vi "AnalogDisc_Core.vi"(8 "error in":errorcluster, 9 "SignalBufferQueue in":refnum<queue>, 10 "DWFCtrlQueue in":refnum<queue>) -> (0 "error out":errorcluster)   [LabVIEW 2013, in "AnalogDiscSDKLv.lvlib"]
uses:
  <instrlib>/AnalogDiscSDKLv/AnalogDiscSDKLv.lvlib
  <instrlib>/AnalogDiscSDKLv/VIs/DWF_AnalogIn_Configurations.ctl
  <instrlib>/AnalogDiscSDKLv/VIs/DWF_AcqMode.ctl
  <instrlib>/AnalogDiscSDKLv/VIs/DWF_Filter.ctl
  <instrlib>/AnalogDiscSDKLv/VIs/DWF_TrigSrc.ctl
  <instrlib>/AnalogDiscSDKLv/VIs/DWF_TrigCond.ctl
  <instrlib>/AnalogDiscSDKLv/VIs/DWF_TrigType.ctl
  <instrlib>/AnalogDiscSDKLv/VIs/DWF_CtrlQueue.ctl
  <instrlib>/AnalogDiscSDKLv/VIs/DWF_State.ctl
  <instrlib>/AnalogDiscSDKLv/VIs/DWF_PrivateStats.ctl
  <instrlib>/AnalogDiscSDKLv/VIs/DWF_InstrumentStatus.ctl
  <instrlib>/AnalogDiscSDKLv/VIs/DWF_DwfState.ctl
  <instrlib>/AnalogDiscSDKLv/VIs/DWF_Signal.ctl
  <instrlib>/AnalogDiscSDKLv/VIs/DWF_TrigLen.ctl
  <instrlib>/AnalogDiscSDKLv/VIs/DWF_DWFERC.ctl
  <vilib>/Utility/error.llb/DialogType.ctl
  <instrlib>/AnalogDiscSDKLv/VIs/DWF_AnalogOut_ChannelConfigurations.ctl
  <instrlib>/AnalogDiscSDKLv/VIs/DWF_Function.ctl
  <instrlib>/AnalogDiscSDKLv/VIs/DWF_Node.ctl
  <vilib>/Utility/miscctls.llb/LVPositionTypeDef.ctl
  <vilib>/Analysis/1siggen.llb/Ramp Pattern by Samples.vi
  <vilib>/Utility/error.llb/Error Cluster From Error Code.vi
  <vilib>/ErrorRing/Error Ring.xnode
  <vilib>/ptbypt/NI_PtbyPt.lvlib
  <userlib>/Utility/ErrorLog_lib.lvlib
  Windows/System32/dwf.dll
  <vilib>/Analysis/NI_AALBase.lvlib
panel:
  out "WaitForVoltageStablize":bool
  in  "GetInfo":bool
  out "psecPosition":dbl
  out "elements":T1[](array[typedef])
  out "sysCount_inPCTrig":i32
  out "PCTrig_counter":i32
  out "AO2_sts":T3=enum."Armed"
  out "AO1_sts":T3=enum."Armed"
  in  "fStart_AO":bool
  in  "SetFuncData_AO":bool
  in  "SetTrigSrc_AO":bool
  in  "SetEnable_AO":bool
  in  "SetConfig_AO":bool
  in  "SetStates_AO":bool
  out "waited t PCTrig":u32
  out "AI_sts":T4
  in  "TriggerPC":bool
  out "Live Stats":T5
  in  "Mode(N/T)":bool caption="Mode"
  out "Graph":sgl[][](graph)
  in  "fConfig":bool
  in  "Reset":bool
  in  "CloseAll":bool
  in  "Close":bool
  in  "Enumerate":bool
  in  "Open":bool
  in  "Quit":bool
  in  "Start":bool
  in  "ConfigAll":bool
  out "UserName":string[](array[string])
  out "SN":string[](array[string])
  out "DevName":string[](array[string])
  out "DeviceID":i32[](array[numeric])
  out "pnDevice":i32
  out "isBusy":i32[](array[numeric])
  out "DeviceVersion":i32[](array[numeric])
  in  "Configurations":T6={"Acqusition"={"Freq(Hz,SampleRate)"=10000000.0, "BufferSize"=8192, "Mode"=enum."Single", "RecordLength(s)"=0.0008192}, "Channels"=[{"Range(V)"=5.0, "Offset(V)"=0.0, "Filter"=enum."Decimate", "Enable"=TRUE}], "Trigger"={"TriggerSource"=enum."None", "Timeout(s)"=0.0, "Holdoff(s)"=1e-06, "Position/Delay(s)"=0.0}, "AnalogTrigger"={"Channel"=0, "Polarity"=enum."Rising", "Type"=enum."Pulse", "Level(V)"=0.0, "Filter"=enum."MinMax", "Hysterisis(V)"=0.0}, "DevSN"="-1"} {"AnalogTrigger"."Channel" format="%#_6p"; "AnalogTrigger"."Hysterisis(V)" format="%#_6p"; "Acqusition"."RecordLength(s)" format="%#_6p"; "Acqusition"."Freq(Hz,SampleRate)" format="%#_6p"; "Acqusition"."BufferSize" min=1 max=16384 step=1; "Trigger"."Position/Delay(s)" format="%#_6p"; "Trigger"."Holdoff(s)" format="%#_6p"}
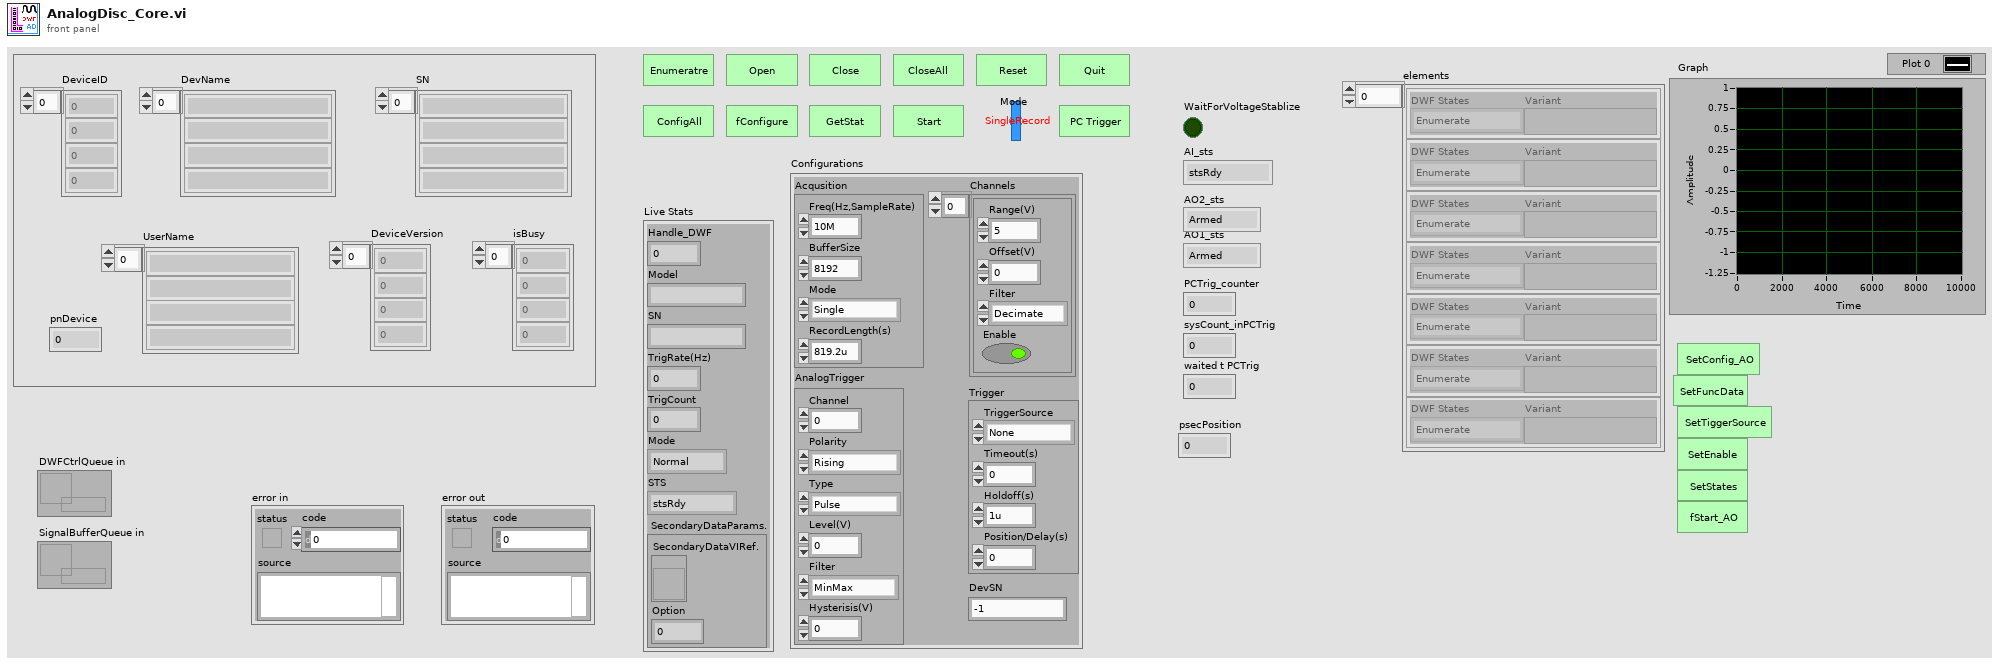
[diagram p1: front panel]
types:
  T1 = typedef "AnalogDiscSDKLv.lvlib/DWF_CtrlQueue.ctl" = cluster{"DWF States":T2, "Variant":variant}
  T2 = typedef "AnalogDiscSDKLv.lvlib/DWF_State.ctl" = enum16{"Enumerate", "Open", "Close", "CloseAll", "Reset", "Quit", "==Settings==", "SetAcquisition_", "SetChannels_", "SetTrigger_", "SetAnalogTrigDetector_", "SetAll_AcquChTrig_", "fConfigurate", "fStart", "GetStatus", "_WaitForDone/Idle", "_GetData", "GetAcquisition", "GetChannels", "GetTrigger", "GetAll_AcquChTrig", "==Messaging==", "_PushDataOut", "GetStat_", "GetConfig_", "==ModeSetup==", "SetSignalBuffer_", "SetMode_", "SetSecondaryDataRef._", "==AnalogOut==", "GetChannelCount_AO", "fStart_AO", "SetChEnable_AO", "SetConfig_AO", "SetFuncData_AO", "SetOffset_AO_", "SetMasterNode_AO", "SetStates_AO", "SetSymetry_AO", "SetTriggerSource_AO", "==Trigger==", "ManualTrigger"}
  T3 = typedef "AnalogDiscSDKLv.lvlib/DWF_DwfState.ctl" = enum16{"Ready", "Armed", "Done", "Running", "Config", "Prefill", "---", "Wait"}
  T4 = typedef "AnalogDiscSDKLv.lvlib/DWF_InstrumentStatus.ctl" = enum16{"stsRdy", "stsARM", "stsDone", "stsTrig", "stsCfg", "stsPrefill", "stsNotDone", "stsTrigDly", "stsError", "stsBusy", "stsStop"}
  T5 = typedef "AnalogDiscSDKLv.lvlib/DWF_PrivateStats.ctl" = cluster{"Handle_DWF":i32, "Model":string, "SN":string, "TrigRate(Hz)":dbl, "TrigCount":i32, "Mode":enum16{"Normal", "Turbo"}, "STS":T4, "SecondaryDataParams.":cluster{"SecondaryDataVIRef.":refnum<vi>, "Option":i32}}
  T6 = typedef "AnalogDiscSDKLv.lvlib/DWF_AnalogIn_Configurations.ctl" = cluster{"Acqusition":cluster{"Freq(Hz,SampleRate)":dbl, "BufferSize":i32, "Mode":T7, "RecordLength(s)":dbl}, "Channels":cluster{"Range(V)":dbl, "Offset(V)":dbl, "Filter":T8, "Enable":bool}[], "Trigger":cluster{"TriggerSource":T9, "Timeout(s)":dbl, "Holdoff(s)":dbl, "Position/Delay(s)":dbl}, "AnalogTrigger":cluster{"Channel":i32, "Polarity":T10, "Type":T11, "Level(V)":dbl, "Filter":T8, "Hysterisis(V)":dbl}, "DevSN":string}
  T7 = typedef "AnalogDiscSDKLv.lvlib/DWF_AcqMode.ctl" = enum16{"Single", "ScanShift", "ScanScreen", "Record"}
  T8 = typedef "AnalogDiscSDKLv.lvlib/DWF_Filter.ctl" = enum16{"Decimate", "Average", "MinMax"}
  T9 = typedef "AnalogDiscSDKLv.lvlib/DWF_TrigSrc.ctl" = enum16{"None", "PC", "DetectorAnalogIn", "DetectorDigitalIn", "AnalogIn", "DigitalIn", "DigitalOut", "AnalogOut1", "AnalogOut2", "AnalogOut3", "AnalogOut4", "External1", "External2", "External3", "External4"}
  T10 = typedef "AnalogDiscSDKLv.lvlib/DWF_TrigCond.ctl" = enum16{"Rising", "Falling"}
  T11 = typedef "AnalogDiscSDKLv.lvlib/DWF_TrigType.ctl" = enum16{"Edge", "Pulse", "Transition"}
  T12 = typedef "LVPositionTypeDef.ctl" = cluster{"Left":i32, "Top":i32}
  T13 = typedef "AnalogDiscSDKLv.lvlib/DWF_AnalogOut_ChannelConfigurations.ctl" = cluster{"FUNC":T14, "Frequency(Hz)_AO":dbl, "Amplitude(V)_AO":dbl, "Phase(deg)_AO":dbl, "Offset(V)_AO":dbl, "rgdData":dbl[], "cData":i32, "Symmetry":dbl, "Enable":bool, "Node":T15}
  T14 = typedef "AnalogDiscSDKLv.lvlib/DWF_Function.ctl" = u8
  T15 = typedef "AnalogDiscSDKLv.lvlib/DWF_Node.ctl" = enum16{"Carrier", "FM", "AM"}
  T16 = cluster{"Configs":T13[], "ChannelCount":i32, "States":cluster{"Wait(s)":dbl, "Run(s)":dbl, "cRepeat":i32, "TriggerSource":T9}[]}
  T17 = typedef "DialogType.ctl" = u16
  T18 = typedef "AnalogDiscSDKLv.lvlib/DWF_DWFERC.ctl" = enum16{"dwfercNoErc", "dwfercUnknownError", "dwfercApiLockTimeout", "dwfercAlreadyOpened", "dwfercNotSupported", "dwfercInvalidParameter0", "dwfercInvalidParameter1", "dwfercInvalidParameter2", "dwfercInvalidParameter3"}
  T19 = typedef "AnalogDiscSDKLv.lvlib/DWF_TrigLen.ctl" = enum16{"triglenLess", "triglenTimeout", "triglenMore"}
  T20 = typedef "AnalogDiscSDKLv.lvlib/DWF_Signal.ctl" = cluster{"tickcount":u32, "Signal":sgl[][], "SecondaryData":dbl[]}
  T21 = cluster{"Freq(Hz,SampleRate)":dbl, "BufferSize":i32, "Mode":T7, "RecordLength(s)":dbl}
  T22 = cluster{"Range(V)":dbl, "Offset(V)":dbl, "Filter":T8, "Enable":bool}[]
  T23 = cluster{"TriggerSource":T9, "Timeout(s)":dbl, "Holdoff(s)":dbl, "Position/Delay(s)":dbl}
  T24 = cluster{"Channel":i32, "Polarity":T10, "Type":T11, "Level(V)":dbl, "Filter":T8, "Hysterisis(V)":dbl}
  T25 = cluster{"SecondaryDataVIRef.":refnum<vi>, "Option":i32}
  T26 = cluster{"Wait(s)":dbl, "Run(s)":dbl, "cRepeat":i32, "TriggerSource":T9}[]
  T27 = cluster{"Wait(s)":dbl, "Run(s)":dbl, "cRepeat":i32, "TriggerSource":T9}
  T28 = cluster{i32, "States":cluster{"Wait(s)":dbl, "Run(s)":dbl, "cRepeat":i32, "TriggerSource":T9}}
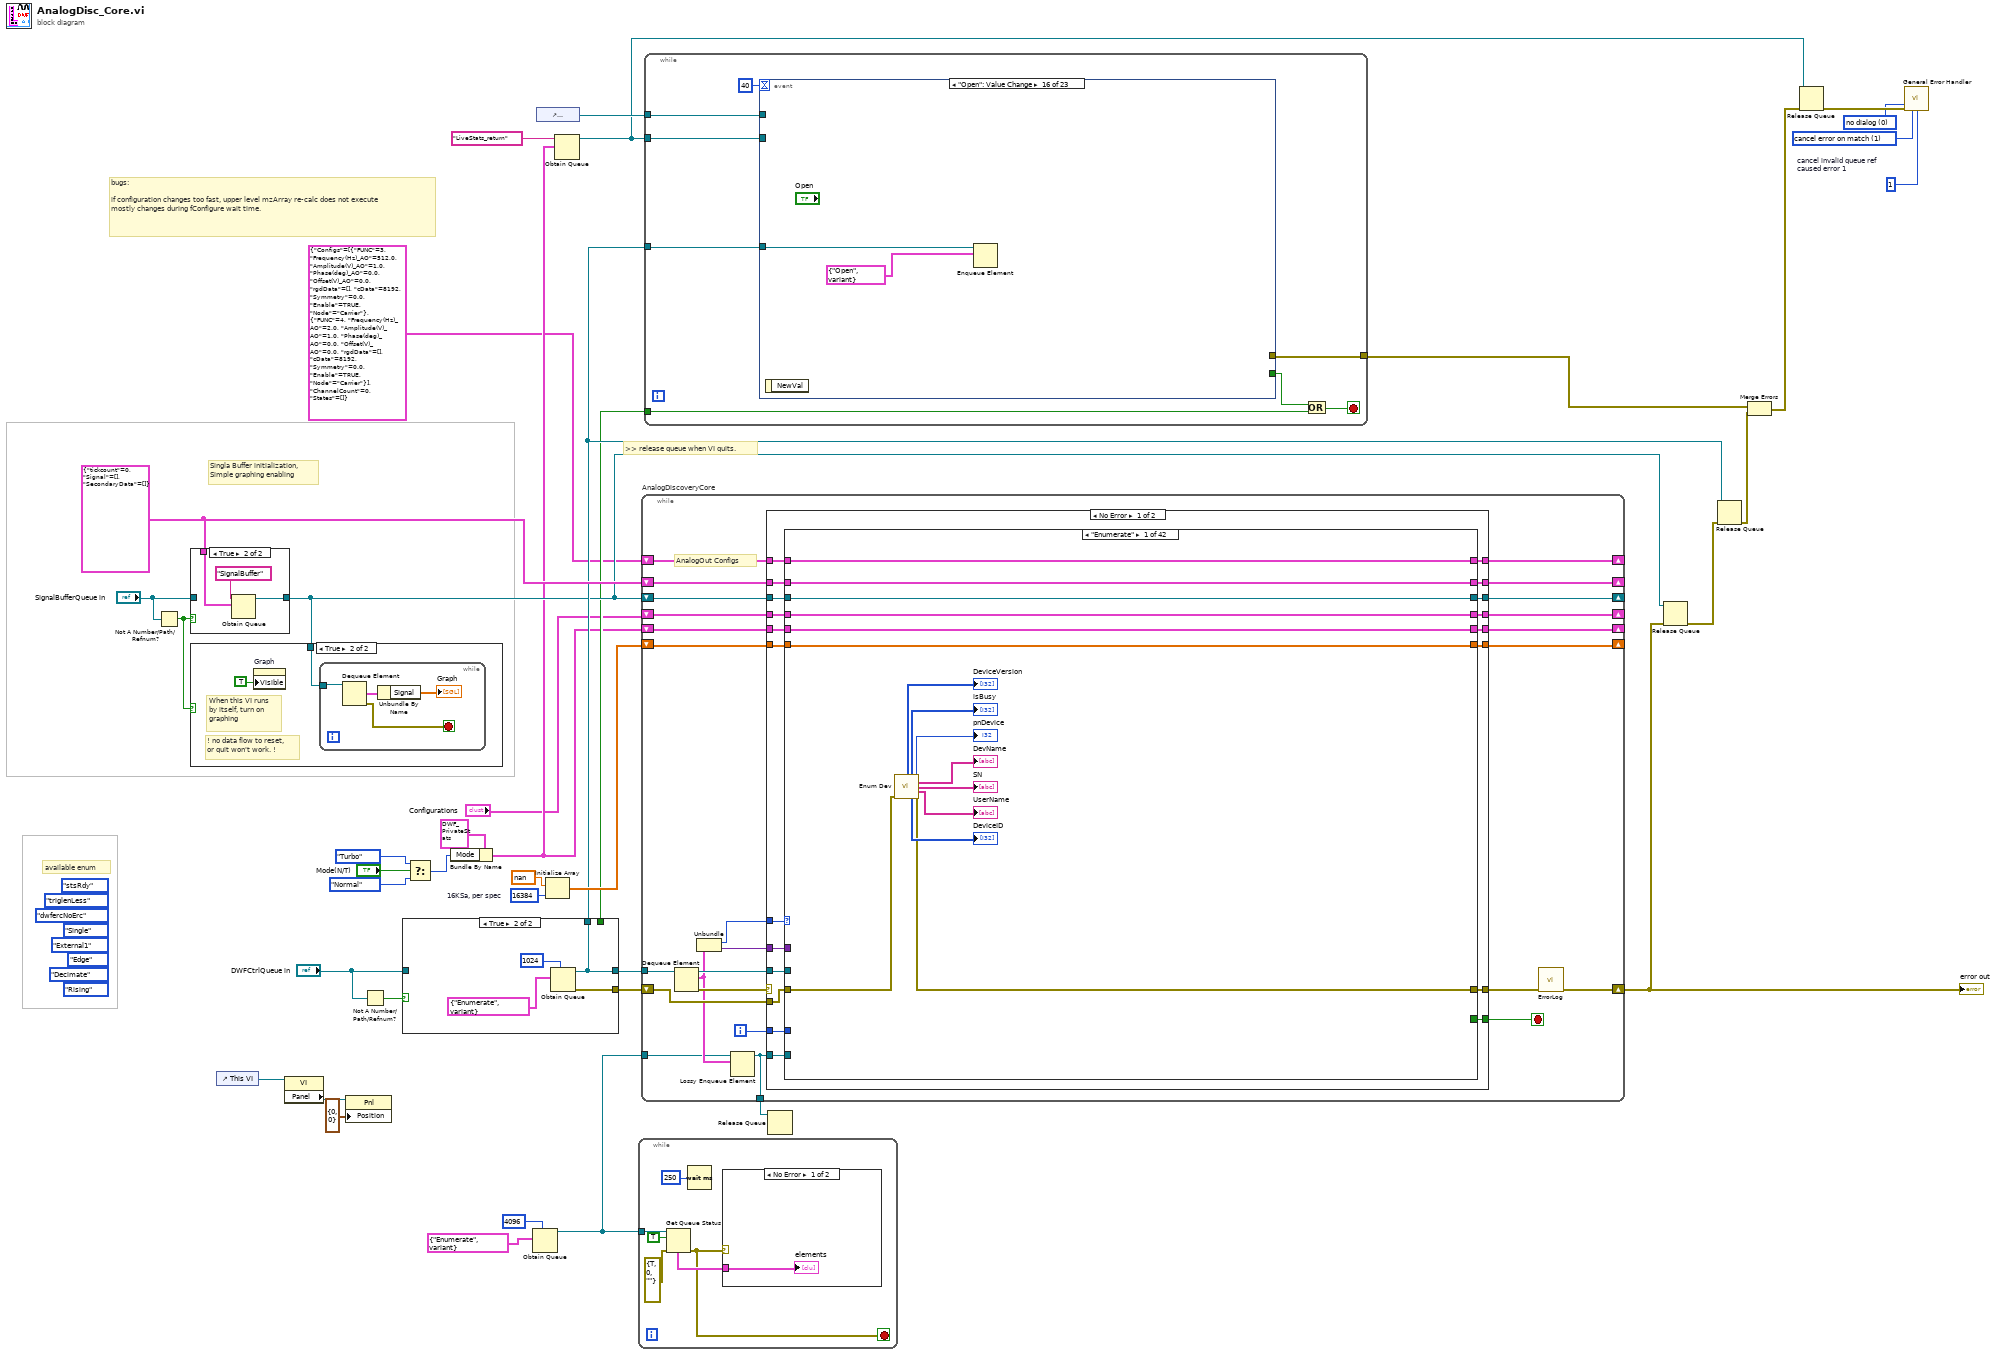
[diagram p0: block diagram]
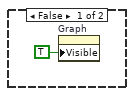
[diagram p3: hidden frame]
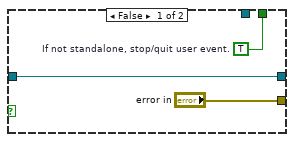
[diagram p5: hidden frame]
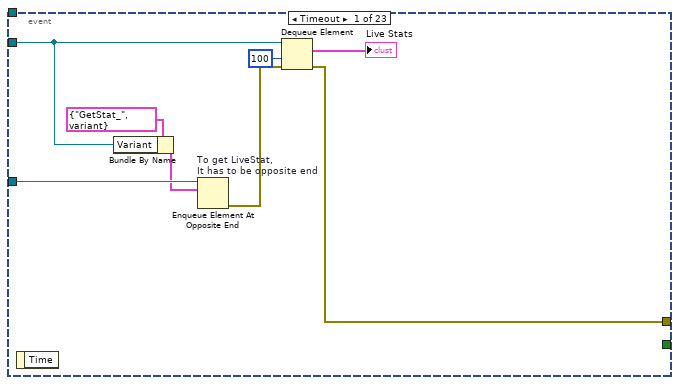
[diagram p6: hidden frame]
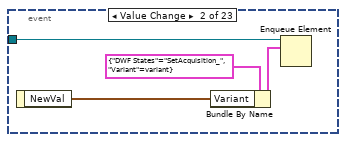
[diagram p7: hidden frame]
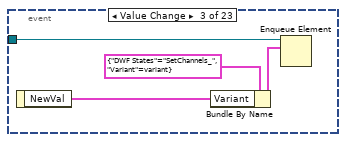
[diagram p8: hidden frame]
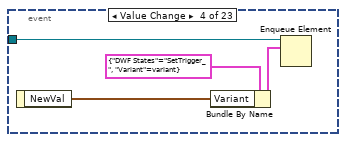
[diagram p9: hidden frame]
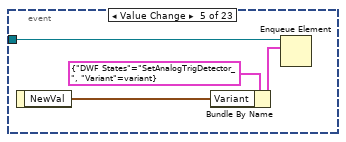
[diagram p10: hidden frame]
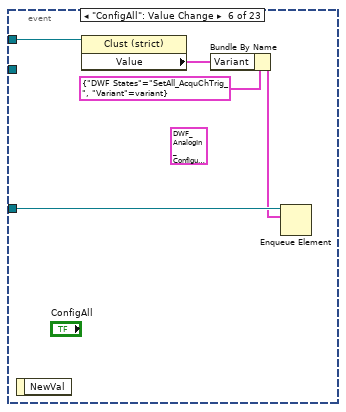
[diagram p11: hidden frame]
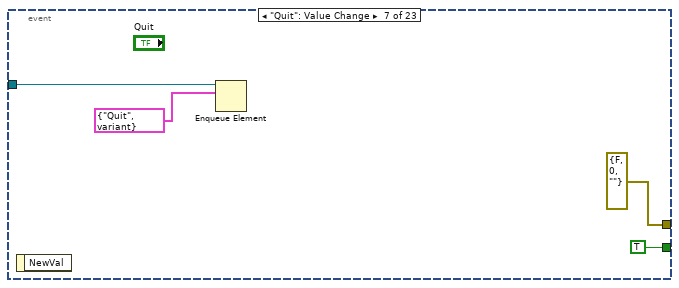
[diagram p12: hidden frame]
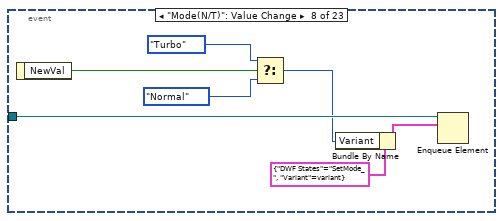
[diagram p13: hidden frame]
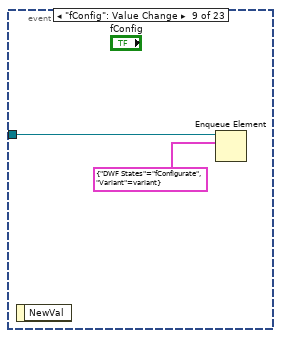
[diagram p14: hidden frame]
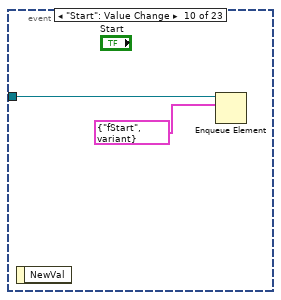
[diagram p15: hidden frame]
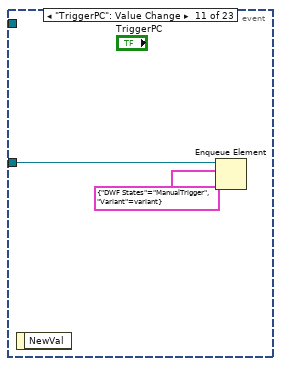
[diagram p16: hidden frame]
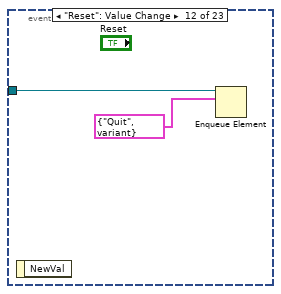
[diagram p17: hidden frame]
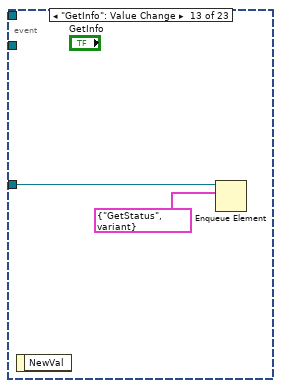
[diagram p18: hidden frame]
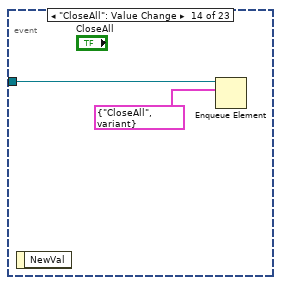
[diagram p19: hidden frame]
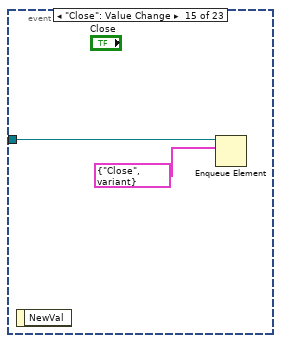
[diagram p20: hidden frame]
diagram:
  w19 = 1  # cancel invalid queue ref caused error 1
  w20 = 1 items=["no exception", "cancel error on match", "set error on match"] ("[exception action] (none:0)")
  w21 = T17 0 items=["no dialog", "OK message", "continue or stop message", "OK message + warnings", "continue/stop + warnings"] ("type of dialog (OK msg:1)")
  (unwired) DWF_TrigSrc."External1" ("TriggerSource")
  (unwired) DWF_DWFERC."dwfercNoErc" ("DWFErC")
  (unwired) DWF_TrigLen."triglenLess" ("TrigLen")
  (unwired) DWF_TrigCond."Rising" ("TrigCond")
  (unwired) DWF_TrigType."Edge" ("TrigType")
  (unwired) DWF_Filter."Decimate" ("Filter")
  (unwired) DWF_AcqMode."Single" ("ACQMODE")
  (unwired) DWF_InstrumentStatus."stsRdy" ("STS")
  w38 = 16384  # 16KSa, per spec
  w40 = T20 {"tickcount"=0, "Signal"=[], "SecondaryData"=[]} ("Signal_Typedef")
  # "bugs:\n\nif configuration changes too fast, upper level mzArray re-calc does not execute\nmostly changes during fConfigure wait time."
  # "Singla Buffer initialization,\nSimple graphing enabling"
  # "available enum"
  # ">> release queue when VI quits."
  n1 = Not A Number/Path/Refnum?(number/path/refnum="SignalBufferQueue in") -> (NaN/Path/Refnum?=w24:bool)
  n2 = case shown="True" w24 {
    tunnel: w40 -> [_ w44]
    tunnel: [w41 w43] -> w25
    tunnel: "SignalBufferQueue in" -> [w41 _]
    frame False {
    }
    frame True {
      n3 = Obtain Queue(name (unnamed)="SignalBuffer", element data type=w44) -> (queue out=w43:refnum<queue>)  [unwired: 3 in, 2 out]
    }
  }
  n4 = case shown="True" w24 {
    tunnel: w25 -> [_ w47]
    frame False {
      n5 = property on="Graph" class="WFGraph (strict)"("Visible"=TRUE) -> ()  [unwired: 2 in, 2 out]
    }
    frame True {
      # "! no data flow to reset,\nor quit won't work. !"
      # "When this VI runs\nby itself, turn on \ngraphing"
      n6 = property on="Graph" class="WFGraph (strict)"("Visible"=TRUE) -> ()  [unwired: 2 in, 2 out]
      n7 = while {
        tunnel: w47 -> [w51]
        stop <- w48 stop-if-true
        n8 = Dequeue Element(queue=w51) -> (element=w50:T20, error out=w48:errorcluster)  [unwired: 2 in, 2 out]
        n9 = Unbundle By Name(w50) -> ("Signal"=→"Graph":sgl[][])
      }
    }
  }
  n10 = control-ref of="This VI"() -> (w3:refnum<vi>)
  n11 = property class="VI"(reference=w3) -> ("Panel"=w2:refnum<vi>)  [unwired: 1 in, 2 out]
  n12 = property class="Pnl"(reference=w2, "Position"=T12 {"Left"=0, "Top"=0}) -> ()  [unwired: 1 in, 2 out]
  n13 = Not A Number/Path/Refnum?(number/path/refnum="DWFCtrlQueue in") -> (NaN/Path/Refnum?=w34:bool)
  n14 = case shown="True" w34 {
    tunnel: [w54 w55] -> w36
    tunnel: ["error in" w58] -> w35
    tunnel: "DWFCtrlQueue in" -> [w54 _]
    tunnel: [_ w55] -> w30
    tunnel: [w52 _] -> w18
    frame False {
      w52 = TRUE  # If not standalone, stop/quit user event.
    }
    frame True {
      n15 = Obtain Queue(max queue size (-1, unlimited)=1024, element data type=T1 {"DWF States"=enum."Enumerate", "Variant"=variant}) -> (queue out=w55:refnum<queue>, error out=w58:errorcluster)  [unwired: 3 in, 1 out]
    }
  }
  n16 = Select(t=enum16{"Normal", "Turbo"}."Turbo" ("Mode"), s="Mode(N/T)", f=enum16{"Normal", "Turbo"}."Normal" ("Mode")) -> (s? t:f=w11:enum16{"Normal", "Turbo"})
  n17 = Bundle By Name(cluster=T5 {"Handle_DWF"=0, "Model"="", "SN"="", "TrigRate(Hz)"=0.0, "TrigCount"=0, "Mode"=enum."Normal", "STS"=enum."stsRdy", "SecondaryDataParams."={"SecondaryDataVIRef."=refnum, "Option"=0}} ("PrivateStats(Live)"), "Mode"=w11) -> (w15:T5)
  n18 = Obtain Queue(max queue size (-1, unlimited)=4096, element data type=T1 {"DWF States"=enum."Enumerate", "Variant"=variant}) -> (queue out=w5:refnum<queue>)  [unwired: 3 in, 2 out]
  n19 = control-ref of="Configurations"() -> (w32:refnum<vi>)
  n20 = Initialize Array(nan ("Numeric"), w38) -> (w37:dbl[])
  n21 = Obtain Queue(name (unnamed)="LiveStats_return", element data type=w15) -> (queue out=w28:refnum<queue>)  [unwired: 3 in, 2 out]
  n22 = while {
    tunnel: w5 -> [w64]
    stop <- w61 stop-if-true
    n23 = Get Queue Status(queue=w64, return elements? (F)=TRUE, error in (no error)=errorcluster {"status"=TRUE, "code"=0, "source"=""}) -> (error out=w61:errorcluster, elements=w62:T1[])  [unwired: 6 out]
    n24 = Wait (ms)(milliseconds to wait=u32 250) -> ()  [unwired: 1 out]
    n25 = case shown="No Error" w61 {
      tunnel: w62 -> [w65 _]
      frame No Error {
        "elements" <- w65
      }
      frame Error {
      }
    }
  }
  n26 = while "AnalogDiscoveryCore" {
    shift-right: [w89] -> _
    shift-left: w25 -> [w90]
    tunnel: w36 -> [w71]
    shift-right: [w70] -> w23
    shift-left: w35 -> [w77]
    shift-right: [w86] -> _
    shift-left: "Configurations" -> [w85]
    shift-right: [w78] -> _
    shift-left: w15 -> [w84]
    shift-right: [w79] -> _
    shift-left: w37 -> [w82]
    shift-right: [w80] -> _
    shift-left: w40 -> [w83]
    shift-right: [w73] -> _
    shift-left: T16 {"Configs"=[{"FUNC"=3, "Frequency(Hz)_AO"=512.0, "Amplitude(V)_AO"=1.0, "Phase(deg)_AO"=0.0, "Offset(V)_AO"=0.0, "rgdData"=[], "cData"=8192, "Symmetry"=0.0, "Enable"=TRUE, "Node"=enum."Carrier"}, {"FUNC"=4, "Frequency(Hz)_AO"=2.0, "Amplitude(V)_AO"=1.0, "Phase(deg)_AO"=0.0, "Offset(V)_AO"=0.0, "rgdData"=[], "cData"=8192, "Symmetry"=0.0, "Enable"=TRUE, "Node"=enum."Carrier"}], "ChannelCount"=0, "States"=[]} -> [w74]
    tunnel: w5 -> [w68]
    tunnel: [w66] -> w4
    i -> [w72]
    stop <- w88 stop-if-true
    # "AnalogOut Configs"
    n27 = Dequeue Element(queue=w71) -> (queue out=w75:refnum<queue>, element=w69:T1, error out=w76:errorcluster)  [unwired: 2 in, 1 out]
    n28 = Unbundle(w69) -> ("DWF States"=w67:T2, "Variant"=w81:variant)
    n29 = Lossy Enqueue Element(queue=w68, element=w69) -> (queue out=w66:refnum<queue>)  [unwired: 1 in, 3 out]
    n30 = case shown="No Error" w76 {
      tunnel: w90 -> [w110 w1205]
      tunnel: [w109 w1205] -> w89
      tunnel: [w108 TRUE] -> w88
      tunnel: [w107 w1203] -> w87
      tunnel: [w106 w1206] -> w86
      tunnel: w85 -> [w105 w1206]
      tunnel: w84 -> [w104 w1207]
      tunnel: w83 -> [w103 w1204]
      tunnel: w82 -> [w102 w1208]
      tunnel: w75 -> [w101 _]
      tunnel: w67 -> [w100 _]
      tunnel: w81 -> [w99 _]
      tunnel: [w98 w1204] -> w80
      tunnel: [w97 w1208] -> w79
      tunnel: [w96 w1207] -> w78
      tunnel: w77 -> [w95 _]
      tunnel: w74 -> [w94 w1202]
      tunnel: [w93 w1202] -> w73
      tunnel: w72 -> [w92 _]
      tunnel: w66 -> [w91 _]
      frame No Error {
        n31 = case shown="\"Enumerate\"" w100 {
          tunnel: w110 -> [w125 w139 w184 w192 w208 w224 w248 w267 w301 w337 w367 w396 w440 w456 w469 w493 w559 w586 w593 w600 w612 w624 w631 w675 w687 w699 w708 w743 w767 w774 w785 w800 w828 w872 w933 w978 w1020 w1069 w1117 w1153 w1160 w1181]
          tunnel: [w125 w139 w184 w192 w208 w224 w248 w267 w301 w337 w367 w396 w440 w456 w469 w493 w559 w586 w593 w600 w612 w624 w631 w675 w687 w699 w708 w744 w767 w774 w785 w800 w828 w872 w933 w978 w1020 w1069 w1117 w1153 w1160 w1181] -> w109
          tunnel: [_ _ _ _ _ w218 _ _ _ _ _ _ _ _ _ _ _ _ _ _ _ _ _ _ _ _ _ _ _ _ _ _ _ _ _ _ _ _ _ _ _ _] -> w108
          tunnel: w101 -> [_ _ _ _ w204 w215 _ _ _ _ _ w392 _ w443 _ w495 w547 _ _ _ _ _ w647 _ _ _ _ _ _ _ _ _ _ _ _ _ _ _ _ _ _ _]
          tunnel: w95 -> [w116 _ w176 w191 w203 w216 _ w258 w292 w329 w360 w386 w433 w447 w463 w494 w545 w585 w592 w599 w602 _ w649 w669 w677 _ w713 w740 w756 w773 w775 w787 w818 w863 w924 w969 w1011 w1060 w1102 w1147 _ w1174]
          tunnel: [w117 w134 w175 w191 w202 w217 w243 w259 w293 w326 w357 w391 w427 w449 w462 w487 w549 w585 w592 w599 w603 w619 w648 w668 w678 w694 w709 w741 w757 w773 w776 w788 w819 w864 w925 w970 w1012 w1061 w1109 w1142 w1154 w1175] -> w107
          tunnel: [w124 w132 w183 w190 w207 w223 w247 w264 w298 w334 w364 w389 w439 w455 w468 w492 w564 w584 w591 w598 w604 w623 w651 w667 w679 w698 w717 w749 w766 w772 w784 w799 w827 w871 w932 w977 w1019 w1068 w1116 w1152 w1159 w1180] -> w106
          tunnel: w105 -> [w124 w132 w183 w190 w207 w223 w247 w262 w296 w332 w362 w389 w439 w455 w468 w492 w564 w584 w591 w598 w604 w623 w651 w667 w679 w698 w717 w749 w766 w772 w784 w799 w827 w871 w932 w977 w1019 w1068 w1116 w1152 w1159 w1180]
          tunnel: [w123 w137 w179 w189 w201 w220 w246 w265 w299 w335 w365 w395 w435 w451 w461 w484 w542 w583 w590 w597 w611 w622 w645 w666 w686 w697 w710 w748 w763 w771 w780 w796 w824 w868 w929 w974 w1016 w1065 w1113 w1149 w1158 w1176] -> w96
          tunnel: w104 -> [w123 w136 w180 w189 w201 w220 w246 w265 w299 w335 w365 w395 w435 w451 w465 w485 w552 w583 w590 w597 w611 w622 w635 w666 w686 w697 w707 w748 w762 w771 w780 w796 w824 w868 w929 w974 w1016 w1065 w1113 w1149 w1158 w1176]
          tunnel: w103 -> [w122 w138 w182 w188 w206 w222 w245 w266 w300 w336 w366 w394 w438 w454 w467 w490 w558 w582 w589 w596 w610 w621 w644 w674 w685 w696 w716 w747 w765 w770 w783 w798 w826 w870 w931 w976 w1018 w1067 w1115 w1151 w1157 w1179]
          tunnel: w102 -> [w115 w135 w177 w187 w205 w221 w244 w255 w290 w327 w358 w393 w432 w445 w466 w486 w563 w581 w588 w595 w609 w620 w646 w673 w684 w695 w715 w746 w764 w769 w782 w797 w825 w869 w930 w975 w1017 w1066 w1114 w1150 w1156 w1178]
          tunnel: w99 -> [_ _ _ _ _ _ _ w263 w297 w333 w363 w390 _ _ _ _ _ _ _ _ w608 _ _ w670 w683 _ w714 w745 w761 _ _ w794 w822 w866 w927 w972 w1014 w1063 w1111 w1148 _ _]
          tunnel: [w122 w138 w182 w188 w206 w222 w245 w266 w300 w336 w366 w394 w438 w454 w467 w490 w557 w582 w589 w596 w610 w621 w644 w674 w685 w696 w716 w747 w765 w770 w783 w798 w826 w870 w931 w976 w1018 w1067 w1115 w1151 w1157 w1179] -> w98
          tunnel: [w115 w135 w177 w187 w205 w221 w244 w256 w290 w327 w358 w393 w432 w445 w466 w486 w543 w581 w588 w595 w609 w620 w646 w673 w684 w695 w715 w746 w764 w769 w782 w797 w825 w869 w930 w975 w1017 w1066 w1114 w1150 w1156 w1178] -> w97
          tunnel: w94 -> [w111 w133 w174 w185 w195 w213 w242 w254 w289 w325 w356 w385 w431 w444 w459 w471 w539 w580 w587 w594 w601 w618 w634 w664 w676 w693 w705 w737 w755 w768 w781 w793 w816 w857 w918 w963 w1005 w1056 w1105 w1141 w1155 w1177]
          tunnel: [w111 w133 w174 w185 w195 w213 w242 w254 w289 w325 w356 w385 w431 w444 w459 w471 w539 w580 w587 w594 w601 w618 w634 w664 w676 w693 w705 w737 w755 w768 w778 w793 w815 w856 w917 w962 w1004 w1055 w1104 w1141 w1155 w1177] -> w93
          tunnel: w92 -> [_ _ _ _ _ _ _ _ _ _ _ _ _ _ _ _ _ _ _ _ _ _ _ _ _ _ _ _ _ _ _ _ _ _ _ _ _ _ _ _ _ w1166]
          tunnel: w91 -> [_ _ _ _ _ _ _ _ _ _ _ _ _ _ _ _ _ _ _ _ _ _ _ _ _ _ _ _ _ _ _ _ _ _ _ _ _ _ _ _ _ _]
          frame "Enumerate" {
            n32 = call <instrlib>:"Enum Dev.vi"("error in (no error)"=w116) -> ("DeviceVersion"=→"DeviceVersion":i32[], "isBusy"=→"isBusy":i32[], "pnDevice"=→"pnDevice":i32, "DevName"=→"DevName":string[], "SN"=→"SN":string[], "UserName"=→"UserName":string[], "DeviceID"=→"DeviceID":i32[], "error out"=w117:errorcluster)  [unwired: 7 in]
          }
          frame "Open" {
            # "if did not fine => -1,\nwhich mean the first\navailable device."
            n33 = Unbundle By Name(w132) -> ("DevSN"=w126:string)
            n34 = call <instrlib>:"Enum Dev.vi"() -> ("DevName"=w129:string[], "SN"=w131:string[], "error out"=w130:errorcluster)  [unwired: 8 in, 5 out]
            n35 = Search 1D Array "find index of the dev by SN"(1D array=w131, element=w126) -> (index of element=w127:i32)  [unwired: 1 in]
            n36 = Less Than 0?(x=w127) -> (x < 0?=w128:bool)
            n37 = case shown="False" w128 {
              tunnel: [w149 w167] -> w137
              tunnel: w136 -> [w148 w167]
              tunnel: [w145 w168] -> w134
              tunnel: w130 -> [w143 _]
              tunnel: w126 -> [w142 _]
              tunnel: w129 -> [w141 _]
              tunnel: w127 -> [w140 _]
              frame False {
                n38 = call <vilib>:"Clear Errors.vi"("error in (no error)"=w143) -> ("error out"=w146:errorcluster)  [unwired: 6 in]
                n39 = call <instrlib>:"Open Dev.vi"("error in (no error)"=w146, "idxDev"=w140) -> ("error out"=w147:errorcluster, "hdwf"=w144:i32)  [unwired: 7 in, 1 out]
                n40 = case shown="No Error" w147 {
                  selector: w147 -> [w153 _]
                  tunnel: [w159 w161] -> w149
                  tunnel: w144 -> [w156 _]
                  tunnel: w148 -> [w155 w161]
                  tunnel: w142 -> [w154 _]
                  tunnel: [w153 w160] -> w145
                  tunnel: w141 -> [w152 _]
                  tunnel: w140 -> [w150 _]
                  frame No Error {
                    n41 = Index Array(array=w152, index=w150) -> (element=w151:string)
                    n42 = Bundle By Name(cluster=w155, "Handle_DWF"=w156, "SN"=w154, "TrigRate(Hz)"=0.0, "TrigCount"=0, "Model"=w151) -> (w159:T5)
                  }
                  frame Error {
                    n43 = xnode "Error Ring"() -> ("error out"=w160:errorcluster)
                  }
                }
              }
              frame True {
                n44 = xnode "Error Ring"() -> ("error out"=w168:errorcluster)
              }
            }
          }
          frame "Close" {
            n45 = Unbundle By Name(w180) -> ("Handle_DWF"=w181:i32)
            n46 = call <instrlib>:"Close Dev.vi"("error in (no error)"=w176, "hdwf"=w181) -> ("error out"=w175:errorcluster)  [unwired: 8 in, 1 out]
            n47 = Bundle By Name(cluster=w180, "Handle_DWF"=-1) -> (w179:T5)
          }
          frame "CloseAll" {
            n48 = for {
              N: 4 -> [_]
              i -> [w194]
              n49 = call <instrlib>:"Close Dev.vi"("hdwf"=w194) -> ("error out"=w193:errorcluster)  [unwired: 9 in, 1 out]
              n50 = call <vilib>:"Clear Errors.vi"("error in (no error)"=w193) -> ()  [unwired: 6 in, 1 out]
            }
          }
          frame "Reset" {
            n51 = Unbundle By Name(w201) -> ("SN"=w199:string)
            n52 = Bundle By Name(cluster=T1 {"DWF States"=enum."Open", "Variant"=variant} ("element"), "Variant"=w199) -> (w198:T1)
            n53 = Build Array(w198, T1 {"DWF States"=enum."Close", "Variant"=variant} ("element")) -> (w196:T1[])
            n54 = for {
              tunnel: w204 -> [w212]
              tunnel: w196 -> [w209] mode=indexing
              shift-right: [w210] -> w202
              shift-left: w203 -> [w211]
              n55 = Enqueue Element At Opposite End(queue=w212, element=w209, error in (no error)=w211) -> (error out=w210:errorcluster)  [unwired: 1 in, 2 out]
            }
          }
          frame "Quit" {
            n56 = Unbundle By Name(w220) -> ("SecondaryDataParams..SecondaryDataVIRef."=w214:refnum<vi>, "Handle_DWF"=w219:i32)
            n57 = case "Check handle leak??" shown="-1" w219 {
              tunnel: [_ TRUE] -> w218
              tunnel: [w226 w235] -> w217
              tunnel: w216 -> [w227 w236]
              tunnel: w215 -> [w228 _]
              tunnel: w214 -> [_ w233]
              frame Default {
                n58 = for {
                  tunnel: w228 -> [w232]
                  tunnel: T1[] [{"DWF States"=enum."Quit", "Variant"=variant}, {"DWF States"=enum."Close", "Variant"=variant}] -> [w229] mode=indexing
                  shift-right: [w230] -> w226
                  shift-left: w227 -> [w231]
                  n59 = Enqueue Element At Opposite End(queue=w232, element=w229, error in (no error)=w231) -> (error out=w230:errorcluster)  [unwired: 1 in, 2 out]
                }
              }
              frame -1 {
                n60 = Not A Number/Path/Refnum?(number/path/refnum=w233) -> (NaN/Path/Refnum?=w234:bool)
                n61 = case shown="False" w234 {
                  tunnel: w233 -> [w240 _]
                  tunnel: w236 -> [w239 w241]
                  tunnel: [w238 w241] -> w235
                  frame False {
                    n62 = Close Reference "Release secondarydatavi Reference"(reference=w240, error in (no error)=w239) -> (error out=w238:errorcluster)
                  }
                  frame True {
                  }
                }
              }
            }
          }
          frame "==Settings==" {
            # "Invalid frame"
            n63 = xnode "Error Ring"() -> ("error out"=w243:errorcluster)
          }
          frame "SetAcquisition_" {
            n64 = Unbundle By Name(w262) -> ("Acqusition"=w261:T21)
            n65 = Variant To Data(error in=w258, type=w261, Variant=w263) -> (data=w260:T21, error out=w257:errorcluster)
            n66 = Bundle By Name(cluster=w262, "Acqusition"=w260) -> (w264:T6)
            n67 = case shown="No Error" w257 {
              selector: w257 -> [w274 _]
              tunnel: w265 -> [w281 _]
              tunnel: w260 -> [w279 _]
              tunnel: [w276 w283] -> w259
              tunnel: [w273 w282] -> w256
              tunnel: w255 -> [_ w282]
              frame No Error {
                n68 = Unbundle By Name(w279) -> ("Mode"=w278:T7, "Freq(Hz,SampleRate)"=w277:dbl, "BufferSize"=w271:i32, "RecordLength(s)"=w268:dbl)
                n69 = Unbundle By Name(w281) -> ("Handle_DWF"=w280:i32)
                n70 = call <instrlib>:"Set Acquisition Config Analog In.vi"("RecordLength(s)"=w268, "AcqMode"=w278, "error in (no error)"=w274, "BufferSize"=w271, "Frquency(MS/s)"=w277, "hdwf"=w280) -> ("error out"=w276:errorcluster)  [unwired: 3 in, 2 out]
                n71 = In Range and Coerce(upper limit=16384, x=w271, lower limit=1) -> (coerced(x)=w272:i32)  [unwired: 1 out]
                n72 = Initialize Array(nan ("Numeric"), w272) -> (w273:dbl[])
              }
              frame Error {
                n73 = xnode "Error Ring"() -> ("error out"=w283:errorcluster)
              }
            }
          }
          frame "SetChannels_" {
            n74 = Unbundle By Name(w296) -> ("Channels"=w295:T22)
            n75 = Variant To Data(error in=w292, type=w295, Variant=w297) -> (data=w294:T22, error out=w291:errorcluster)
            n76 = Bundle By Name(cluster=w296, "Channels"=w294) -> (w298:T6)
            n77 = case shown="No Error" w291 {
              selector: w291 -> [w302 _]
              tunnel: w299 -> [w306 _]
              tunnel: w294 -> [w304 _]
              tunnel: [w303 w317] -> w293
              frame No Error {
                n78 = Unbundle By Name(w306) -> ("Handle_DWF"=w305:i32)
                n79 = for {
                  tunnel: w305 -> [w316]
                  tunnel: w304 -> [w315] mode=indexing
                  shift-right: [w308] -> w303
                  shift-left: w302 -> [w307]
                  i -> [w309]
                  n80 = Unbundle By Name(w315) -> ("Offset(V)"=w313:dbl, "Range(V)"=w314:dbl, "Enable"=w311:bool, "Filter"=w312:T8)
                  n81 = Boolean To (0,1)(Boolean=w311) -> (0, 1=w310:i16)
                  n82 = call <instrlib>:"Set Channels Config Analog In.vi"("voltOffset"=w313, "Filter"=w312, "voltsRange"=w314, "error in (no error)"=w307, "Enable"=w310, "indexCh"=w309, "hdwf"=w316) -> ("error out"=w308:errorcluster)  [unwired: 2 in, 2 out]
                }
              }
              frame Error {
                n83 = xnode "Error Ring"() -> ("error out"=w317:errorcluster)
              }
            }
          }
          frame "SetTrigger_" {
            n84 = Unbundle By Name(w332) -> ("Trigger"=w331:T23)
            n85 = Variant To Data(error in=w329, type=w331, Variant=w333) -> (data=w330:T23, error out=w328:errorcluster)
            n86 = Bundle By Name(cluster=w332, "Trigger"=w330) -> (w334:T6)
            n87 = case shown="No Error" w328 {
              selector: w328 -> [w346 _]
              tunnel: w335 -> [w348 _]
              tunnel: w330 -> [w347 _]
              tunnel: [w342 w349] -> w326
              tunnel: [w341 _] -> w324
              tunnel: [w340 _] -> w323
              frame No Error {
                n88 = Unbundle By Name(w347) -> ("Timeout(s)"=w345:dbl, "TriggerSource"=w343:T9, "Position/Delay(s)"=w340:dbl, "Holdoff(s)"=w344:dbl)
                n89 = Unbundle By Name(w348) -> ("Handle_DWF"=w341:i32)
                n90 = call <instrlib>:"Set Analog In Trigger.vi"("secHoldOff"=w344, "secPosition"=w340, "secTimeout"=w345, "error in (no error)"=w346, "trigsrc"=w343, "hdwf"=w341) -> ("error out"=w342:errorcluster)  [unwired: 4 in, 1 out]
              }
              frame Error {
                n91 = xnode "Error Ring"() -> ("error out"=w349:errorcluster)
              }
            }
            n92 = disable-structure shown="Disabled" {
              disable-tunnel: w324 -> [w339 _]
              disable-tunnel: w323 -> [w338 _]
              frame Disabled {
                n93 = dll-call lib="C:/Windows/System32/dwf.dll" fn="FDwfAnalogInTriggerPositionSet"("hdwf"=w339, "secPosition"=w338) -> ()  [unwired: 6 in, 2 out]
              }
              frame Enabled {
              }
            }
          }
          frame "SetAnalogTrigDetector_" {
            n94 = Unbundle By Name(w362) -> ("AnalogTrigger"=w355:T24)
            n95 = Variant To Data(error in=w360, type=w355, Variant=w363) -> (data=w361:T24, error out=w359:errorcluster)
            n96 = Bundle By Name(cluster=w362, "AnalogTrigger"=w361) -> (w364:T6)
            n97 = case shown="No Error" w359 {
              selector: w359 -> [w377 _]
              tunnel: w365 -> [w378 _]
              tunnel: w361 -> [w368 _]
              tunnel: [w376 w379] -> w357
              frame No Error {
                n98 = Unbundle By Name(w378) -> ("Handle_DWF"=w375:i32)
                n99 = Unbundle By Name(w368) -> ("Hysterisis(V)"=w374:dbl, "Level(V)"=w373:dbl, "Channel"=w372:i32, "Polarity"=w371:T10, "Type"=w370:T11, "Filter"=w369:T8)
                n100 = call <instrlib>:"Set Analog In Trigger Detector.vi"("hdwf"=w375, "voltsLevel"=w373, "HystersisvoltsLevel"=w374, "idxChannel"=w372, "trigcond"=w371, "trigtype"=w370, "error in (no error)"=w377, "filter"=w369) -> ("error out"=w376:errorcluster)  [unwired: 6 in, 1 out]
              }
              frame Error {
                n101 = xnode "Error Ring"() -> ("error out"=w379:errorcluster)
              }
            }
          }
          frame "SetAll_AcquChTrig_" {
            n102 = Variant To Data(type=w389, Variant=w390) -> (data=w387:T6, error out=w388:errorcluster)  [unwired: 1 in]
            n103 = case shown="No Error" w388 {
              tunnel: w392 -> [w414 _]
              tunnel: [w413 w419] -> w391
              tunnel: w387 -> [w412 _]
              tunnel: w386 -> [w411 _]
              frame No Error {
                n104 = Unbundle By Name(w412) -> ("Acqusition"=w409:T21, "Channels"=w407:T22, "Trigger"=w405:T23, "AnalogTrigger"=w399:T24)
                n105 = Bundle By Name(cluster=T1 {"DWF States"=enum."SetAcquisition_", "Variant"=variant} ("element"), "Variant"=w409) -> (w404:T1)
                n106 = Bundle By Name(cluster=T1 {"DWF States"=enum."SetChannels_", "Variant"=variant} ("element"), "Variant"=w407) -> (w403:T1)
                n107 = Bundle By Name(cluster=T1 {"DWF States"=enum."SetTrigger_", "Variant"=variant} ("element"), "Variant"=w405) -> (w402:T1)
                n108 = Bundle By Name(cluster=T1 {"DWF States"=enum."SetAnalogTrigDetector_", "Variant"=variant} ("element"), "Variant"=w399) -> (w398:T1)
                n109 = Build Array(w404, w403, w402, w398) -> (w401:T1[])
                n110 = Reverse 1D Array(array=w401) -> (reversed array=w397:T1[])
                n111 = for {
                  tunnel: w414 -> [w418]
                  shift-right: [w417] -> w413
                  shift-left: w411 -> [w416]
                  tunnel: w397 -> [w415] mode=indexing
                  n112 = Enqueue Element At Opposite End(queue=w418, element=w415, error in (no error)=w416) -> (error out=w417:errorcluster)  [unwired: 1 in, 2 out]
                }
              }
              frame Error {
                n113 = xnode "Error Ring"() -> ("error out"=w419:errorcluster)
              }
            }
          }
          frame "fConfigurate" {
            n114 = Unbundle By Name(w435) -> ("Handle_DWF"=w434:i32)
            n115 = call <instrlib>:"Config Analog In.vi"("error in (no error)"=w433, "fStart"=0, "fReconfigure"=1, "hdwf"=w434) -> ("error out"=w430:errorcluster)  [unwired: 5 in, 2 out]
            n116 = property on="WaitForVoltageStablize" class="Bool (strict)"(error in=w430, "Value"=TRUE ("WaitForVoltageStablize")) -> (error out=w429:errorcluster)  [unwired: 1 in, 1 out]
            n117 = flat-sequence {
              tunnel: [w441] -> w428
              tunnel: w429 -> [w441]
              frame #0 {
                # "todo:\nSend Out message: \nWaiting for offest voltage stablized."
                n118 = Wait (ms) "Wait for voltage stablize \n(According to SDK manual)"(milliseconds to wait=u32 1500) -> ()  [unwired: 1 out]
              }
            }
            n119 = property on="WaitForVoltageStablize" class="Bool (strict)"(error in=w428, "Value"=FALSE ("WaitForVoltageStablize")) -> (error out=w427:errorcluster)  [unwired: 1 in, 1 out]
          }
          frame "fStart" {
            n120 = Unbundle By Name(w451) -> ("Handle_DWF"=w450:i32)
            n121 = Enqueue Element(queue=w443, element=T1 {"DWF States"=enum."_WaitForDone/Idle", "Variant"=variant}, error in (no error)=w447) -> (error out=w446:errorcluster)  [unwired: 1 in, 2 out]
            n122 = call <instrlib>:"Config Analog In.vi"("error in (no error)"=w446, "fStart"=1, "fReconfigure"=0, "hdwf"=w450) -> ("error out"=w449:errorcluster)  [unwired: 5 in, 2 out]
          }
          frame "GetStatus" {
            n123 = Unbundle By Name(w465) -> ("Handle_DWF"=w458:i32)
            n124 = call <instrlib>:"Get Status Analog In.vi"("error in (no error)"=w463, "fReadData"=0, "hdwf"=w458) -> ("error out"=w462:errorcluster, "psts"=w460:T4)  [unwired: 5 in, 1 out]
            n125 = Bundle By Name(cluster=w465, "STS"=w460) -> (w461:T5)
            n126 = dll-call lib="C:/Windows/System32/dwf.dll" fn="FDwfAnalogInTriggerPositionGet"("hdwf"=w458) -> ("psecPosition"=→"psecPosition":dbl)  [unwired: 6 in, 2 out]
          }
          frame "_WaitForDone/Idle" {
            w479 = T2[] [enum."Close", enum."CloseAll", enum."Reset", enum."Quit", enum."GetStatus"] items=["Enumerate", "Open", "Close", "CloseAll", "Reset", "Quit", "==Settings==", "SetAcquisition_", "SetChannels_", "SetTrigger_", "SetAnalogTrigDetector_", "SetAll_AcquChTrig_", "fConfigurate", "fStart", "GetStatus", "_WaitForDone/Idle", "_GetData", "GetAcquisition", "GetChannels", "GetTrigger", "GetAll_AcquChTrig", "==Messaging==", "_PushDataOut", "GetStat_", "GetConfig_", "==ModeSetup==", "SetSignalBuffer_", "SetMode_", "SetSecondaryDataRef._", "==AnalogOut==", "GetChannelCount_AO", "fStart_AO", "SetChEnable_AO", "SetConfig_AO", "SetFuncData_AO", "SetOffset_AO_", "SetMasterNode_AO", "SetStates_AO", "SetSymetry_AO", "SetTriggerSource_AO", "==Trigger==", "ManualTrigger"]
            # "Logic:\nClose => Quit\ntimeout =>"
            n127 = Unbundle By Name(w485) -> ("SecondaryDataParams..SecondaryDataVIRef."=w473:refnum<vi>, "SecondaryDataParams..Option"=w472:i32, "Handle_DWF"=w491:i32)
            n128 = Wait Until Next ms Multiple(millisecond multiple=u32 1) -> ()  [unwired: 1 out]
            n129 = call <instrlib>:"Get Status Analog In.vi"("error in (no error)"=w494, "hdwf"=w491) -> ("error out"=w476:errorcluster, "psts"=w474:T4)  [unwired: 6 in, 1 out]
            n130 = Preview Queue Element(queue=w495, timeout in ms (-1)=0, error in (no error)=w476) -> (queue out=w489:refnum<queue>, element=w482:T1, timed out?=w480:bool, error out=w488:errorcluster)
            n131 = Bundle By Name(cluster=w485, "STS"=w474) -> (w484:T5)
            n132 = Unbundle(w482) -> ("DWF States"=w470:T2)  [unwired: 1 out]
            n133 = Search 1D Array(1D array=w479, element=w470) -> (index of element=w478:i32)  [unwired: 1 in]
            n134 = Greater Or Equal To 0?(x=w478) -> (x >= 0?=w477:bool)
            n135 = Compound Arithmetic op=AND(w477, invert w480) -> (w475:bool)
            n136 = case shown="False" w475 {
              tunnel: w489 -> [w501 _]
              tunnel: w488 -> [w500 w534]
              tunnel: [w499 w534] -> w487
              tunnel: w474 -> [w498 _]
              tunnel: w473 -> [w497 _]
              tunnel: w472 -> [w496 _]
              tunnel: w470 -> [_ _]
              frame False {
                # "queue empty OR other command"
                n137 = case shown="\"stsRdy\"" w498 {
                  tunnel: w501 -> [w502 w516 _ w528]
                  tunnel: w500 -> [w505 w514 w525 w527]
                  tunnel: [w504 w515 w525 w526] -> w499
                  tunnel: w497 -> [_ w510 _ _]
                  tunnel: w496 -> [_ w513 _ _]
                  frame "stsRdy" {
                    # "Typically, this is caused by config change\nduring acquisition. \nPush fConfig and fStart to continure  acuisition."
                    n138 = for {
                      shift-right: [w508] -> w504
                      shift-left: w505 -> [w509]
                      tunnel: T1[] [{"DWF States"=enum."fConfigurate", "Variant"=variant}, {"DWF States"=enum."fStart", "Variant"=variant}] -> [w507] mode=indexing
                      tunnel: w502 -> [w506]
                      n139 = Enqueue Element(queue=w506, element=w507, error in (no error)=w509) -> (error out=w508:errorcluster)  [unwired: 1 in, 2 out]
                    }
                  }
                  frame "stsDone" {
                    n140 = Not A Number/Path/Refnum?(number/path/refnum=w510) -> (NaN/Path/Refnum?=w511:bool)
                    n141 = case shown="True" w511 {
                      tunnel: w510 -> [w520 _]
                      tunnel: w514 -> [w519 w521]
                      tunnel: w513 -> [w518 _]
                      tunnel: [w517 w521] -> w512
                      frame False {
                        n142 = call-by-ref "Maybe this give a little bit \nbetter timing precision\nfor secondary data?"(reference=w520, error in=w519, "Index"=w518) -> (error out=w517:errorcluster)  [unwired: 10 in, 2 out]
                      }
                      frame True {
                      }
                    }
                    n143 = flat-sequence {
                      tunnel: w516 -> [w524]
                      tunnel: [w522] -> w515
                      tunnel: w512 -> [w522]
                      frame #0 {
                        n144 = Enqueue Element(queue=w524, element=T1 {"DWF States"=enum."_GetData", "Variant"=variant}) -> ()  [unwired: 2 in, 3 out]
                      }
                    }
                  }
                  frame "stsError", "stsStop" {
                  }
                  frame Default {
                    n145 = disable-structure "Driven by outter layer queue timeout" shown="Enabled" {
                      disable-tunnel: w528 -> [w532 _]
                      disable-tunnel: w527 -> [w531 w533]
                      disable-tunnel: [w530 w533] -> w526
                      frame Enabled {
                        n146 = Enqueue Element(queue=w532, element=T1 {"DWF States"=enum."_WaitForDone/Idle", "Variant"=variant}, error in (no error)=w531) -> (error out=w530:errorcluster)  [unwired: 1 in, 2 out]
                      }
                      frame Disabled {
                      }
                    }
                  }
                }
              }
              frame True {
              }
            }
          }
          frame "_GetData" {
            # "If 0 channel enabled, then this should generate\n an empty array output in queue"
            n147 = Unbundle By Name(w552) -> ("TrigCount"=w540:i32, "Handle_DWF"=w551:i32, "Mode"=w548:enum16{"Normal", "Turbo"})
            n148 = Unbundle By Name(w564) -> ("Acqusition.Freq(Hz,SampleRate)"=w538:dbl, "Acqusition.RecordLength(s)"=w537:dbl, "Acqusition.BufferSize"=w535:i32, "Channels"=w561:T22)
            n149 = Enqueue Element(queue=w547, element=T1 {"DWF States"=enum."_PushDataOut", "Variant"=variant}, error in (no error)=w545) -> (error out=w544:errorcluster)  [unwired: 1 in, 2 out]
            n150 = Tick Count (ms)() -> (millisecond timer value=w562:u32)
            n151 = Array Size(array=w561) -> (size(s)=w560:i32)
            n152 = Multiply(x=w538, y=w537) -> (x*y=w536:dbl)
            n153 = Round To Nearest(number=w536) -> ()  [unwired: 1 out]
            n154 = for {
              N: w560 -> [_]
              tunnel: [w573] -> w555 mode=indexing
              tunnel: w535 -> [w579]
              shift-right: [w573] -> w543
              shift-left: w563 -> [w577]
              tunnel: [w575] -> w556
              tunnel: w562 -> [w575]
              shift-right: [w574] -> w553
              shift-left: w544 -> [w576]
              shift-right: [w571] -> w550
              shift-left: w551 -> [w572]
              i -> [w578]
              n155 = call <instrlib>:"Get Data Analog In.vi"("BufferSize"=w579, "error in (no error)"=w576, "rgdSamples"=w577, "idxChannel"=w578, "hdwf"=w572) -> ("error out"=w574:errorcluster, "rgdSamples out"=w573:dbl[], "function return"=w571:i32)  [unwired: 4 in]
            }
            n156 = Increment(x=w540) -> (x+1=w541:i32)
            n157 = To Single Precision Float(number=w555) -> (single precision float=w554:sgl[][])
            n158 = Bundle By Name(cluster=w552, "TrigCount"=w541) -> (w542:T5)
            n159 = Bundle By Name(cluster=w558, "tickcount"=w556, "Signal"=w554) -> (w557:T20)
            n160 = case shown="\"Turbo\"" w548 {
              tunnel: w553 -> [w565 w570]
              tunnel: w550 -> [_ w569]
              tunnel: [w565 w568] -> w549
              frame "Normal", Default {
              }
              frame "Turbo" {
                n161 = call <instrlib>:"Config Analog In.vi"("error in (no error)"=w570, "fStart"=1, "fReconfigure"=0, "hdwf"=w569) -> ("error out"=w568:errorcluster)  [unwired: 5 in, 2 out]
              }
            }
          }
          frame "GetAcquisition" {
          }
          frame "GetChannels" {
          }
          frame "GetTrigger" {
          }
          frame "GetAll_AcquChTrig" {
            n162 = Variant To Data(type=refnum<queue> refnum ("queue out"), Variant=w608) -> (data=w606:refnum<queue>, error out=w605:errorcluster)  [unwired: 1 in]
            n163 = case shown="No Error" w605 {
              selector: w605 -> [_ w617]
              tunnel: w606 -> [w616 _]
              tunnel: w604 -> [w615 _]
              tunnel: [w614 w617] -> w603
              tunnel: w602 -> [w613 _]
              frame No Error {
                # "short term solution, need refine\nget real result from device"
                n164 = Enqueue Element(queue=w616, element=w615, error in (no error)=w613) -> (error out=w614:errorcluster)  [unwired: 1 in, 2 out]
              }
              frame Error {
              }
            }
          }
          frame "==Messaging==" {
            # "Invalid Frame"
            n165 = xnode "Error Ring"() -> ("error out"=w619:errorcluster)
          }
          frame "_PushDataOut" {
            n166 = Unbundle By Name(w635) -> ("SecondaryDataParams..SecondaryDataVIRef."=w632:refnum<vi>)
            n167 = Unbundle By Name(w635) -> ("Mode"=w650:enum16{"Normal", "Turbo"})
            n168 = case "Actually, does NOTHING." shown="\"Turbo\"" w650 {
              tunnel: w649 -> [w657 w663]
              tunnel: [w657 w662] -> w648
              tunnel: w647 -> [_ w661]
              frame "Normal" {
              }
              frame "Turbo" {
                # "In turbo mode, \nre-arming is done in \"_GetData\"\n\nNormal mode => no need to re-arming  daq"
                n169 = Enqueue Element(queue=w661, element=T1 {"DWF States"=enum."_WaitForDone/Idle", "Variant"=variant}, error in (no error)=w663) -> (queue out=w659:refnum<queue>, error out=w662:errorcluster)  [unwired: 1 in, 1 out]
                n170 = Enqueue Element(queue=w659, element=T1 {"DWF States"=enum."ManualTrigger", "Variant"=variant}) -> ()  [unwired: 2 in, 3 out]
              }
            }
            n171 = Not A Number/Path/Refnum?(number/path/refnum=w632) -> (NaN/Path/Refnum?=w633:bool)
            n172 = case shown="False" w633 {
              tunnel: w644 -> [w655 w656]
              tunnel: w632 -> [w654 _]
              tunnel: [w652 w656] -> w630
              frame False {
                n173 = call-by-ref "Get SecondaryData"(reference=w654) -> ("SecondaryData"=w653:dbl[])  [unwired: 12 in, 2 out]
                n174 = Bundle By Name(cluster=w655, "SecondaryData"=w653) -> (w652:T20)
              }
              frame True {
              }
            }
            n175 = Enqueue Element "Send/Push Data Out"(queue=w631, element=w630) -> ()  [unwired: 2 in, 3 out]
            n176 = Unbundle By Name(w644) -> ("tickcount"=w639:u32)
            n177 = Tick Count (ms)() -> (millisecond timer value=w643:u32)
            n178 = feedback #1(w643) -> (w642:u32)
            n179 = feedback-in #1(w639) -> ()
            n180 = Subtract(x=w639, y=w642) -> (x-y=w640:u32)
            n181 = Divide(x=1000.0, y=w640) -> (x/y=w637:dbl)
            n182 = call <vilib>:"Mean PtByPt.vi"("x"=w637, "sample length"=16) -> ("mean"=w638:dbl)  [unwired: 2 in, 1 out]
            n183 = Bundle By Name(cluster=w635, "TrigRate(Hz)"=w638) -> (w645:T5)
          }
          frame "GetStat_" {
            n184 = Variant To Data(error in=w669, type=refnum<queue> refnum ("queue out"), Variant=w670) -> (data=w672:refnum<queue>, error out=w671:errorcluster)
            n185 = Enqueue Element "Send Core Stat"(queue=w672, element=w666, error in (no error)=w671) -> (error out=w668:errorcluster)  [unwired: 1 in, 2 out]
          }
          frame "GetConfig_" {
            # "solution:\n\n1 call vi ref, vi send out typed command. => possible, idea, time consuming \n\n2 make this frame specific, bad. \n\n3 user event call and wait, then send typed command.  possible, fast?"
            n186 = Variant To Data(type=refnum<queue> refnum ("queue out"), Variant=w683) -> (data=w681:refnum<queue>, error out=w680:errorcluster)  [unwired: 1 in]
            n187 = case shown="No Error" w680 {
              selector: w680 -> [_ w692]
              tunnel: w681 -> [w691 _]
              tunnel: w679 -> [w690 _]
              tunnel: [w689 w692] -> w678
              tunnel: w677 -> [w688 _]
              frame No Error {
                # "short term solution, need refine\nget real result from device"
                n188 = Enqueue Element(queue=w691, element=w690, error in (no error)=w688) -> (error out=w689:errorcluster)  [unwired: 1 in, 2 out]
              }
              frame Error {
              }
            }
          }
          frame "==ModeSetup==" {
            # "Invalid Frame"
            n189 = xnode "Error Ring"() -> ("error out"=w694:errorcluster)
          }
          frame "SetSecondaryDataRef._" {
            n190 = Unbundle By Name(w707) -> ("SecondaryDataParams."=w706:T25)
            n191 = Variant To Data(error in=w713, type=w706, Variant=w714) -> (data=w711:T25, error out=w712:errorcluster)
            n192 = case shown="No Error" w712 {
              tunnel: w711 -> [w721 _]
              tunnel: w707 -> [w729 w731]
              tunnel: [w728 w731] -> w710
              tunnel: [_ w730] -> w709
              tunnel: w706 -> [w722 _]
              frame No Error {
                n193 = Unbundle By Name(w722) -> ("SecondaryDataVIRef."=w719:refnum<vi>)
                n194 = Unbundle By Name(w721) -> ("Option"=w718:i32, "SecondaryDataVIRef."=w720:refnum<vi>)
                n195 = property class="VI Interface Type 0"(reference=w720) -> (reference out=w725:refnum<vi>, "Path"=w727:path)  [unwired: 1 in, 1 out]
                n196 = Close Reference(reference=w719) -> (error out=w723:errorcluster)  [unwired: 1 in]
                n197 = call <vilib>:"Clear Errors.vi"("error in (no error)"=w723) -> ()  [unwired: 6 in, 1 out]
                n198 = Open VI Reference(type specifier VI Refnum (for type only)=w725, vi path=w727, options=256) -> (vi reference=w724:refnum<vi>)  [unwired: 3 in, 1 out]
                n199 = Bundle By Name(cluster=w729, "SecondaryDataParams..Option"=w718, "SecondaryDataParams..SecondaryDataVIRef."=w724) -> (w728:T5)
              }
              frame Error {
                n200 = xnode "Error Ring"() -> ("error out"=w730:errorcluster)
              }
            }
          }
          frame "SetSignalBuffer_" {
            n201 = Variant To Data(type=w743, Variant=w745) -> (data=w742:refnum<queue>, error out=w739:errorcluster)  [unwired: 1 in]
            n202 = Select(t=w743, s=w739, f=w742) -> (s? t:f=w744:refnum<queue>)
            n203 = xnode "Error Ring"() -> ("error out"=w738:errorcluster)
            n204 = Select(t=w738, s=w739, f=w740) -> (s? t:f=w741:errorcluster)
          }
          frame "SetMode_" {
            n205 = Unbundle By Name(w762) -> ("Mode"=w759:enum16{"Normal", "Turbo"})
            n206 = Variant To Data(error in=w756, type=w759, Variant=w761) -> (data=w758:enum16{"Normal", "Turbo"}, error out=w757:errorcluster)
            n207 = Select(t=w759, s=w757, f=w758) -> (s? t:f=w760:enum16{"Normal", "Turbo"})
            n208 = Bundle By Name(cluster=w762, "Mode"=w760) -> (w763:T5)
          }
          frame "==AnalogOut==" {
          }
          frame "GetChannelCount_AO" {
            n209 = Unbundle By Name(w780) -> ("Handle_DWF"=w779:i32)
            n210 = call <instrlib>:"Get Channel Count Analog Out.vi"("error in (no error)"=w775, "hdwf"=w779) -> ("error out"=w776:errorcluster, "pcChannel"=w777:i32)  [unwired: 7 in, 1 out]
            n211 = Bundle By Name(cluster=w781, "ChannelCount"=w777) -> (w778:T16)
          }
          frame "fStart_AO" {
            n212 = Unbundle By Name(w796) -> ("Handle_DWF"=w795:i32)
            n213 = Bundle(0, 0) -> (w790:cluster{i32, i32})  [unwired: 1 in]
            n214 = Variant To Data(error in=w787, type=w790, Variant=w794) -> (data=w789:cluster{i32, i32}, error out=w786:errorcluster)
            n215 = case shown="No Error" w786 {
              selector: w786 -> [w801 _]
              tunnel: w795 -> [w806 _]
              tunnel: w789 -> [w805 _]
              tunnel: [w802 w807] -> w788
              frame No Error {
                n216 = Unbundle(w805) -> (w804:i32, w803:i32)
                n217 = call <instrlib>:"fStart Analog Out.vi"("error in (no error)"=w801, "fStart"=w803, "idxChannel"=w804, "hdwf"=w806) -> ("error out"=w802:errorcluster)  [unwired: 6 in, 1 out]
              }
              frame Error {
                n218 = xnode "Error Ring"() -> ("error out"=w807:errorcluster)
              }
            }
          }
          frame "SetChEnable_AO" {
            n219 = Unbundle By Name(w824) -> ("Handle_DWF"=w823:i32)
            n220 = Bundle(0, TRUE) -> (w821:cluster{i32, bool})  [unwired: 1 in]
            n221 = Variant To Data(error in=w818, type=w821, Variant=w822) -> (data=w820:cluster{i32, bool}, error out=w817:errorcluster)
            n222 = case shown="No Error" w817 {
              selector: w817 -> [w836 _]
              tunnel: w823 -> [w837 _]
              tunnel: w820 -> [w833 _]
              tunnel: [w832 w850] -> w819
              tunnel: w816 -> [w835 w849]
              tunnel: [w831 w849] -> w815
              frame No Error {
                n223 = Unbundle(w833) -> (w829:i32, w830:bool)
                n224 = in-place {
                  in-place-border: [w841] -> w834
                  in-place-border: w830 -> [w840]
                  in-place-border: w829 -> [w838]
                  n225 = in-place-cluster #2(w835) -> ("Configs"=w842:T13[])
                  n226 = in-place {
                    in-place-border: [w845] -> w841
                    in-place-border: w840 -> [w844]
                    n227 = in-place-array #3(w842, w838) -> (w846:T13)
                    n228 = in-place {
                      in-place-border: [w847] -> w845
                      in-place-border: w844 -> [w848]
                      n229 = in-place-cluster #4(w846) -> ("Node"=w847:T15)  [unwired: 1 out]
                      n230 = in-place-cluster #4("Enable"=w848, "Node"=w847) -> (w843:T13)
                    }
                    n231 = in-place-array #3(w843) -> (w839:T13[])  [unwired: 1 out]
                  }
                  n232 = in-place-cluster #2("Configs"=w839) -> (w831:T16)
                }
                n233 = call <instrlib>:"Set Channel Enable Analog Out.vi"("fEnable"=w830, "error in (no error)"=w836, "node"=w834, "idxChannel"=w829, "hdwf"=w837) -> ("error out"=w832:errorcluster)  [unwired: 6 in]
              }
              frame Error {
                n234 = xnode "Error Ring"() -> ("error out"=w850:errorcluster)
              }
            }
          }
          frame "SetConfig_AO" {
            n235 = Unbundle By Name(w857) -> ("Configs"=w861:T13[])
            n236 = Unbundle By Name(w868) -> ("Handle_DWF"=w867:i32)
            n237 = Index Array(array=w861) -> (element=w860:T13)  [unwired: 1 in]
            n238 = Bundle(0, w860) -> (w858:cluster{i32, T13})  [unwired: 1 in]
            n239 = Variant To Data(error in=w863, type=w858, Variant=w866) -> (data=w865:cluster{i32, T13}, error out=w862:errorcluster)
            n240 = case shown="No Error" w862 {
              selector: w862 -> [w885 _]
              tunnel: w867 -> [w882 _]
              tunnel: w865 -> [w884 _]
              tunnel: [w881 w911] -> w864
              tunnel: w857 -> [w886 w910]
              tunnel: [w873 w910] -> w856
              frame No Error {
                n241 = Unbundle(w884) -> (w880:i32, w883:T13)
                n242 = Unbundle By Name(w883) -> ("Phase(deg)_AO"=w879:dbl, "Amplitude(V)_AO"=w878:dbl, "Node"=w877:T15, "Frequency(Hz)_AO"=w876:dbl, "Offset(V)_AO"=w875:dbl, "FUNC"=w874:T14)
                n243 = in-place {
                  in-place-border: w880 -> [w894]
                  in-place-border: w879 -> [w893]
                  in-place-border: w878 -> [w892]
                  in-place-border: w877 -> [w891]
                  in-place-border: w876 -> [w890]
                  in-place-border: w875 -> [w889]
                  in-place-border: w874 -> [w888]
                  n244 = in-place-cluster #5(w886) -> ("Configs"=w895:T13[])
                  n245 = in-place {
                    in-place-border: w893 -> [w902]
                    in-place-border: w892 -> [w901]
                    in-place-border: w891 -> [w900]
                    in-place-border: w890 -> [w899]
                    in-place-border: w889 -> [w898]
                    in-place-border: w888 -> [w897]
                    n246 = in-place-array #6(w895, w894) -> (w903:T13)
                    n247 = in-place {
                      in-place-border: w902 -> [w909]
                      in-place-border: w901 -> [w908]
                      in-place-border: w900 -> [w907]
                      in-place-border: w899 -> [w906]
                      in-place-border: w898 -> [w905]
                      in-place-border: w897 -> [w904]
                      n248 = in-place-cluster #7(w903) -> ()  [unwired: 6 out]
                      n249 = in-place-cluster #7("Phase(deg)_AO"=w909, "Amplitude(V)_AO"=w908, "Node"=w907, "Frequency(Hz)_AO"=w906, "Offset(V)_AO"=w905, "FUNC"=w904) -> (w896:T13)
                    }
                    n250 = in-place-array #6(w896) -> (w887:T13[])  [unwired: 1 out]
                  }
                  n251 = in-place-cluster #5("Configs"=w887) -> (w873:T16)
                }
                n252 = call <instrlib>:"Set Config Analog Out.vi"("hdwf"=w882, "vAmplitude"=w878, "degPhase"=w879, "idxChannel"=w880, "node"=w877, "hzFrequency"=w876, "error in (no error)"=w885, "vOffset"=w875, "func"=w874) -> ("error out"=w881:errorcluster)  [unwired: 5 in, 1 out]
              }
              frame Error {
                n253 = xnode "Error Ring"() -> ("error out"=w911:errorcluster)
              }
            }
          }
          frame "SetOffset_AO_" {
            n254 = Unbundle By Name(w918) -> ("Configs"=w922:T13[])
            n255 = Unbundle By Name(w929) -> ("Handle_DWF"=w928:i32)
            n256 = Index Array(array=w922) -> (element=w921:T13)  [unwired: 1 in]
            n257 = Bundle(0, w921) -> (w919:cluster{i32, T13})  [unwired: 1 in]
            n258 = Variant To Data(error in=w924, type=w919, Variant=w927) -> (data=w926:cluster{i32, T13}, error out=w923:errorcluster)
            n259 = case shown="No Error" w923 {
              selector: w923 -> [w935 _]
              tunnel: w928 -> [w940 _]
              tunnel: w926 -> [w942 _]
              tunnel: [w934 w956] -> w925
              tunnel: w918 -> [w943 w955]
              tunnel: [w941 w955] -> w917
              frame No Error {
                n260 = Unbundle(w942) -> (w939:i32, w937:T13)
                n261 = Unbundle By Name(w937) -> ("Offset(V)_AO"=w936:dbl)
                n262 = in-place {
                  in-place-border: w939 -> [w947]
                  in-place-border: [w945] -> w938
                  in-place-border: w936 -> [w944]
                  n263 = in-place-cluster #8(w943) -> ("Configs"=w948:T13[])
                  n264 = in-place {
                    in-place-border: [w950] -> w945
                    in-place-border: w944 -> [w949]
                    n265 = in-place-array #9(w948, w947) -> (w952:T13)
                    n266 = in-place {
                      in-place-border: [w953] -> w950
                      in-place-border: w949 -> [w954]
                      n267 = in-place-cluster #10(w952) -> ("Node"=w953:T15)  [unwired: 1 out]
                      n268 = in-place-cluster #10("Offset(V)_AO"=w954, "Node"=w953) -> (w951:T13)
                    }
                    n269 = in-place-array #9(w951) -> (w946:T13[])  [unwired: 1 out]
                  }
                  n270 = in-place-cluster #8("Configs"=w946) -> (w941:T16)
                }
                n271 = dll-call lib="C:/Windows/System32/dwf.dll" fn="FDwfAnalogOutNodeOffsetSet"(error in=w935, "hdwf"=w940, "idxChannel"=w939, "node"=w938, "vOffset"=w936) -> (error out=w934:errorcluster)  [unwired: 7 in, 1 out]
              }
              frame Error {
                n272 = xnode "Error Ring"() -> ("error out"=w956:errorcluster)
              }
            }
          }
          frame "SetSymetry_AO" {
            n273 = Unbundle By Name(w963) -> ("Configs"=w967:T13[])
            n274 = Unbundle By Name(w974) -> ("Handle_DWF"=w973:i32)
            n275 = Index Array(array=w967) -> (element=w966:T13)  [unwired: 1 in]
            n276 = Bundle(0, w966) -> (w964:cluster{i32, T13})  [unwired: 1 in]
            n277 = Variant To Data(error in=w969, type=w964, Variant=w972) -> (data=w971:cluster{i32, T13}, error out=w968:errorcluster)
            n278 = case shown="No Error" w968 {
              selector: w968 -> [w987 _]
              tunnel: w973 -> [w984 _]
              tunnel: w971 -> [w986 _]
              tunnel: [w983 w998] -> w970
              tunnel: w963 -> [w988 w997]
              tunnel: [w980 w997] -> w962
              frame No Error {
                n279 = Unbundle(w986) -> (w982:i32, w985:T13)
                n280 = Unbundle By Name(w985) -> ("Symmetry"=w979:dbl, "Node"=w981:T15)
                n281 = in-place {
                  in-place-border: w982 -> [w991]
                  in-place-border: w979 -> [w989]
                  n282 = in-place-cluster #11(w988) -> ("Configs"=w992:T13[])
                  n283 = in-place {
                    in-place-border: w989 -> [w994]
                    n284 = in-place-array #12(w992, w991) -> (w995:T13)
                    n285 = in-place {
                      in-place-border: w994 -> [w996]
                      n286 = in-place-cluster #13(w995) -> ()  [unwired: 1 out]
                      n287 = in-place-cluster #13("Symmetry"=w996) -> (w993:T13)
                    }
                    n288 = in-place-array #12(w993) -> (w990:T13[])  [unwired: 1 out]
                  }
                  n289 = in-place-cluster #11("Configs"=w990) -> (w980:T16)
                }
                n290 = call <instrlib>:"Set Symmetry Analog Out.vi"("percentageSymmetry"=w979, "error in (no error)"=w987, "node"=w981, "idxChannel"=w982, "hdwf"=w984) -> ("error out"=w983:errorcluster)  [unwired: 5 in, 1 out]
              }
              frame Error {
                n291 = xnode "Error Ring"() -> ("error out"=w998:errorcluster)
              }
            }
          }
          frame "SetFuncData_AO" {
            n292 = Unbundle By Name(w1005) -> ("Configs"=w1009:T13[])
            n293 = Unbundle By Name(w1016) -> ("Handle_DWF"=w1015:i32)
            n294 = Index Array(array=w1009) -> (element=w1008:T13)  [unwired: 1 in]
            n295 = Bundle(0, w1008) -> (w1006:cluster{i32, T13})  [unwired: 1 in]
            n296 = Variant To Data(error in=w1011, type=w1006, Variant=w1014) -> (data=w1013:cluster{i32, T13}, error out=w1010:errorcluster)
            n297 = case shown="No Error" w1010 {
              selector: w1010 -> [w1030 _]
              tunnel: w1015 -> [w1027 _]
              tunnel: w1013 -> [w1029 _]
              tunnel: [w1026 w1047] -> w1012
              tunnel: w1005 -> [w1031 w1046]
              tunnel: [w1024 w1046] -> w1004
              frame No Error {
                n298 = Unbundle(w1029) -> (w1025:i32, w1028:T13)
                n299 = Unbundle By Name(w1028) -> ("rgdData"=w1022:dbl[], "cData"=w1021:i32)
                n300 = in-place {
                  in-place-border: w1025 -> [w1036]
                  in-place-border: [w1035] -> w1023
                  in-place-border: w1022 -> [w1034]
                  in-place-border: w1021 -> [w1033]
                  n301 = in-place-cluster #14(w1031) -> ("Configs"=w1037:T13[])
                  n302 = in-place {
                    in-place-border: [w1041] -> w1035
                    in-place-border: w1034 -> [w1040]
                    in-place-border: w1033 -> [w1039]
                    n303 = in-place-array #15(w1037, w1036) -> (w1042:T13)
                    n304 = in-place {
                      in-place-border: [w1045] -> w1041
                      in-place-border: w1040 -> [w1044]
                      in-place-border: w1039 -> [w1043]
                      n305 = in-place-cluster #16(w1042) -> ("Node"=w1045:T15)  [unwired: 2 out]
                      n306 = in-place-cluster #16("Node"=w1045, "rgdData"=w1044, "cData"=w1043) -> (w1038:T13)
                    }
                    n307 = in-place-array #15(w1038) -> (w1032:T13[])  [unwired: 1 out]
                  }
                  n308 = in-place-cluster #14("Configs"=w1032) -> (w1024:T16)
                }
                n309 = call <instrlib>:"Set Function Data Analog Out.vi"("cdData"=w1021, "rgdData"=w1022, "error in (no error)"=w1030, "node"=w1023, "idxChannel"=w1025, "hdwf"=w1027) -> ("error out"=w1026:errorcluster)  [unwired: 4 in, 1 out]
              }
              frame Error {
                n310 = xnode "Error Ring"() -> ("error out"=w1047:errorcluster)
              }
            }
          }
          frame "SetStates_AO" {
            n311 = Unbundle By Name(w1056) -> ("States"=w1054:T26)
            n312 = Unbundle By Name(w1065) -> ("Handle_DWF"=w1064:i32)
            n313 = Index Array(array=w1054) -> (element=w1053:T27)  [unwired: 1 in]
            n314 = Bundle(0, "States"=w1053) -> (w1057:T28)  [unwired: 1 in]
            n315 = Variant To Data(error in=w1060, type=w1057, Variant=w1063) -> (data=w1062:T28, error out=w1059:errorcluster)
            n316 = case shown="No Error" w1059 {
              selector: w1059 -> [w1079 _]
              tunnel: w1064 -> [w1078 _]
              tunnel: w1062 -> [w1075 _]
              tunnel: [w1077 w1096] -> w1061
              tunnel: w1056 -> [w1080 w1095]
              tunnel: [w1076 w1095] -> w1055
              frame No Error {
                n317 = Unbundle(w1075) -> (w1073:i32, "States"=w1074:T27)
                n318 = Unbundle By Name(w1074) -> ("Run(s)"=w1070:dbl, "Wait(s)"=w1071:dbl, "cRepeat"=w1072:i32)
                n319 = in-place {
                  in-place-border: w1073 -> [w1085]
                  in-place-border: w1072 -> [w1084]
                  in-place-border: w1071 -> [w1083]
                  in-place-border: w1070 -> [w1082]
                  n320 = in-place-cluster #17(w1080) -> ("States"=w1086:T26)
                  n321 = in-place {
                    in-place-border: w1084 -> [w1090]
                    in-place-border: w1083 -> [w1089]
                    in-place-border: w1082 -> [w1088]
                    n322 = in-place-array #18(w1086, w1085) -> (w1091:T27)
                    n323 = in-place {
                      in-place-border: w1090 -> [w1094]
                      in-place-border: w1089 -> [w1093]
                      in-place-border: w1088 -> [w1092]
                      n324 = in-place-cluster #19(w1091) -> ()  [unwired: 3 out]
                      n325 = in-place-cluster #19("Run(s)"=w1092, "Wait(s)"=w1093, "cRepeat"=w1094) -> (w1087:T27)
                    }
                    n326 = in-place-array #18(w1087) -> (w1081:T26)  [unwired: 1 out]
                  }
                  n327 = in-place-cluster #17("States"=w1081) -> (w1076:T16)
                }
                n328 = call <instrlib>:"Set States Analog Out.vi"("cRepeat"=w1072, "secRun"=w1070, "error in (no error)"=w1079, "secWait"=w1071, "idxChannel"=w1073, "hdwf"=w1078) -> ("error out"=w1077:errorcluster)  [unwired: 4 in, 1 out]
              }
              frame Error {
                n329 = xnode "Error Ring"() -> ("error out"=w1096:errorcluster)
              }
            }
          }
          frame "SetTriggerSource_AO" {
            n330 = Unbundle By Name(w1113) -> ("Handle_DWF"=w1112:i32)
            n331 = Bundle(0, "TriggerSource"=DWF_TrigSrc."None") -> (w1106:cluster{i32, "TriggerSource":T9})  [unwired: 1 in]
            n332 = Variant To Data(error in=w1102, type=w1106, Variant=w1111) -> (data=w1110:cluster{i32, "TriggerSource":T9}, error out=w1108:errorcluster)
            n333 = case shown="No Error" w1108 {
              selector: w1108 -> [w1124 _]
              tunnel: w1112 -> [w1123 _]
              tunnel: w1110 -> [w1120 _]
              tunnel: [w1122 w1135] -> w1109
              tunnel: w1105 -> [w1125 w1134]
              tunnel: [w1121 w1134] -> w1104
              frame No Error {
                n334 = Unbundle(w1120) -> (w1119:i32, "TriggerSource"=w1118:T9)
                n335 = in-place {
                  in-place-border: w1119 -> [w1128]
                  in-place-border: w1118 -> [w1127]
                  n336 = in-place-cluster #20(w1125) -> ("States"=w1129:T26)
                  n337 = in-place {
                    in-place-border: w1127 -> [w1131]
                    n338 = in-place-array #21(w1129, w1128) -> (w1132:T27)
                    n339 = in-place {
                      in-place-border: w1131 -> [w1133]
                      n340 = in-place-cluster #22(w1132) -> ()  [unwired: 1 out]
                      n341 = in-place-cluster #22("TriggerSource"=w1133) -> (w1130:T27)
                    }
                    n342 = in-place-array #21(w1130) -> (w1126:T26)  [unwired: 1 out]
                  }
                  n343 = in-place-cluster #20("States"=w1126) -> (w1121:T16)
                }
                n344 = call <instrlib>:"Set Trigger Source Analog Out.vi"("error in (no error)"=w1124, "trigsrc"=w1118, "idxChannel"=w1119, "hdwf"=w1123) -> ("error out"=w1122:errorcluster)  [unwired: 6 in, 1 out]
              }
              frame Error {
                n345 = xnode "Error Ring"() -> ("error out"=w1135:errorcluster)
              }
            }
          }
          frame "SetMasterNode_AO" {
            # "no implemented yet"
            n346 = Unbundle By Name(w1141) -> ("Configs"=w1146:T13[])
            n347 = Unbundle By Name(w1149) -> ()  [unwired: 1 out]
            n348 = Index Array(array=w1146) -> (element=w1145:T13)  [unwired: 1 in]
            n349 = Bundle(0, w1145) -> (w1143:cluster{i32, T13})  [unwired: 1 in]
            n350 = Variant To Data(error in=w1147, type=w1143, Variant=w1148) -> (error out=w1142:errorcluster)  [unwired: 1 out]
          }
          frame "==Trigger==" {
            n351 = xnode "Error Ring"() -> ("error out"=w1154:errorcluster)
          }
          frame "ManualTrigger" {
            # "add: skip manual trigger if timeout, popup notif. timeout"
            n352 = Unbundle By Name(w1176) -> ("Handle_DWF"=w1173:i32)
            n353 = Tick Count (ms)() -> (millisecond timer value=w1171:u32)
            n354 = for {
              N: 500 -> [_]
              tunnel: w1173 -> [w1186]
              tunnel: [w1185] -> w1172
              tunnel: [w1195] -> w1170
              tunnel: w1171 -> [w1194]
              tunnel: [w1194] -> w1169
              i -> [w1191]
              stop <- w1192 stop-if-true
              w1182 = DWF_DwfState."Done" ("AO1_sts")
              n355 = call <instrlib>:"Get Status Analog In.vi"("hdwf"=w1186) -> ("psts"=w1197:T4, "hdwf out"=w1185:i32)  [unwired: 7 in, 1 out]
              "AI_sts" <- w1197
              n356 = Wait (ms)(milliseconds to wait=u32 1) -> ()  [unwired: 1 out]
              n357 = for {
                N: 2 -> [_]
                tunnel: [w1201] -> w1188 mode=indexing
                tunnel: w1185 -> [w1200]
                i -> [w1199]
                n358 = dll-call lib="C:/Windows/System32/dwf.dll" fn="FDwfAnalogOutStatus"("hdwf"=w1200, "idxChannel"=w1199) -> ("psts"=w1201:i32)  [unwired: 7 in, 2 out]
              }
              n359 = Not Equal?(x=w1197, y=DWF_InstrumentStatus."stsPrefill") -> (x != y?=w1193:bool)
              n360 = Index Array(array=w1188) -> (element #1=w1183:i32, element #2=w1187:i32)  [unwired: 2 in]
              "AO1_sts" <- w1183
              "AO2_sts" <- w1187
              n361 = Less Or Equal?(x=w1183, y=w1182) -> (x <= y?=w1189:bool)
              n362 = Less Or Equal?(x=w1187, y=w1182) -> (x <= y?=w1190:bool)
              n363 = Compound Arithmetic op=AND "AI+AO_Armed"(w1193, w1189, w1190) -> (w1192:bool)
              n364 = Tick Count (ms)() -> (millisecond timer value=w1195:u32)
              "PCTrig_counter" <- w1191
            }
            n365 = Subtract(x=w1170, y=w1169) -> (x-y=→"waited t PCTrig":u32)
            n366 = dll-call lib="C:/Windows/System32/dwf.dll" fn="FDwfDeviceTriggerPC"(error in=w1174, "hdwf"=w1172) -> (error out=w1175:errorcluster)  [unwired: 4 in, 1 out]
            "sysCount_inPCTrig" <- w1166
          }
        }
      }
      frame Error {
        n367 = xnode "Error Ring"() -> ("error out"=w1203:errorcluster)
      }
    }
    n368 = call <userlib>:"ErrorLog.vi"("error in (no error)"=w87) -> ("error out"=w70:errorcluster)  [unwired: 10 in]
  }
  "error out" <- w23
  n369 = while {
    tunnel: w30 -> [w1222]
    tunnel: w32 -> [w1221]
    tunnel: w28 -> [w1219]
    tunnel: w18 -> [w1216]
    tunnel: [w1215] -> w16
    stop <- w1217 stop-if-true
    n370 = event shown="[15] \"Open\": Value Change" {
      selector: _ -> [_ _ _ _ _ _ _ _ _ _ _ _ _ _ _ _ _ _ _ _ _ _ _]
      dyn-events: _ -> [_ _ _ _ _ _ _ _ _ _ _ _ _ _ _ _ _ _ _ _ _ _ _]
      timeout: 40 -> [_ _ _ _ _ _ _ _ _ _ _ _ _ _ _ _ _ _ _ _ _ _ _]
      tunnel: w1222 -> [w1230 w1234 w1238 w1242 w1246 w1251 w1255 w1262 w1264 w1266 w1268 w1270 w1272 w1274 w1276 w1278 w1280 w1290 w1303 w1309 w1315 w1330 w1338]
      tunnel: w1221 -> [_ _ _ _ _ w1248 _ _ _ _ _ _ _ _ _ _ _ _ _ _ _ _ _]
      tunnel: w1219 -> [w1229 _ _ _ _ _ _ _ _ _ _ _ _ _ _ _ _ _ _ _ _ _ _]
      tunnel: [_ _ _ _ _ _ TRUE _ _ _ _ _ _ _ _ _ _ _ _ _ _ _ _] -> w1218
      tunnel: [w1228 _ _ _ _ _ errorcluster {"status"=FALSE, "code"=0, "source"=""} ("error constant") _ _ _ _ _ _ _ _ _ _ _ _ _ _ _ _] -> w1215
      event Timeout {
        n371 = event-data() -> ()  [unwired: 1 in, 1 out]
        n372 = Bundle By Name(cluster=T1 {"DWF States"=enum."GetStat_", "Variant"=variant} ("element"), "Variant"=w1229) -> (w1226:T1)
        n373 = Enqueue Element At Opposite End "To get LiveStat,\nIt has to be opposite end"(queue=w1230, element=w1226) -> (error out=w1225:errorcluster)  [unwired: 2 in, 2 out]
        n374 = Dequeue Element(queue=w1229, timeout in ms (-1)=100, error in (no error)=w1225) -> (element=→"Live Stats":T5, error out=w1228:errorcluster)  [unwired: 2 out]
      }
      event Value Change {
        n375 = event-data() -> ("NewVal"=w1231:T21)  [unwired: 1 in]
        n376 = Bundle By Name(cluster=T1 {"DWF States"=enum."SetAcquisition_", "Variant"=variant} ("element"), "Variant"=w1231) -> (w1232:T1)
        n377 = Enqueue Element(queue=w1234, element=w1232) -> ()  [unwired: 2 in, 3 out]
      }
      event Value Change {
        n378 = event-data() -> ("NewVal"=w1235:T22)  [unwired: 1 in]
        n379 = Bundle By Name(cluster=T1 {"DWF States"=enum."SetChannels_", "Variant"=variant} ("element"), "Variant"=w1235) -> (w1236:T1)
        n380 = Enqueue Element(queue=w1238, element=w1236) -> ()  [unwired: 2 in, 3 out]
      }
      event Value Change {
        n381 = event-data() -> ("NewVal"=w1239:T23)  [unwired: 1 in]
        n382 = Bundle By Name(cluster=T1 {"DWF States"=enum."SetTrigger_", "Variant"=variant} ("element"), "Variant"=w1239) -> (w1240:T1)
        n383 = Enqueue Element(queue=w1242, element=w1240) -> ()  [unwired: 2 in, 3 out]
      }
      event Value Change {
        n384 = event-data() -> ("NewVal"=w1243:T24)  [unwired: 1 in]
        n385 = Bundle By Name(cluster=T1 {"DWF States"=enum."SetAnalogTrigDetector_", "Variant"=variant} ("element"), "Variant"=w1243) -> (w1244:T1)
        n386 = Enqueue Element(queue=w1246, element=w1244) -> ()  [unwired: 2 in, 3 out]
      }
      event "ConfigAll": Value Change {
        (unwired) T6 {"Acqusition"={"Freq(Hz,SampleRate)"=100000000.0, "BufferSize"=8192, "Mode"=enum."Single", "RecordLength(s)"=0.0}, "Channels"=[{"Range(V)"=5.0, "Offset(V)"=0.0, "Filter"=enum."Decimate", "Enable"=TRUE}], "Trigger"={"TriggerSource"=enum."None", "Timeout(s)"=0.0, "Holdoff(s)"=0.0, "Position/Delay(s)"=0.0}, "AnalogTrigger"={"Channel"=0, "Polarity"=enum."Rising", "Type"=enum."Pulse", "Level(V)"=0.0, "Filter"=enum."Decimate", "Hysterisis(V)"=0.0}, "DevSN"=""} ("Configurations")
        n387 = event-data() -> ()  [unwired: 1 in, 1 out]
        n388 = property class="Clust (strict)"(reference=w1248) -> ("Value"=w1247:T6)  [unwired: 1 in, 2 out]
        n389 = Bundle By Name(cluster=T1 {"DWF States"=enum."SetAll_AcquChTrig_", "Variant"=variant} ("element"), "Variant"=w1247) -> (w1249:T1)
        n390 = Enqueue Element(queue=w1251, element=w1249) -> ()  [unwired: 2 in, 3 out]
      }
      event "Quit": Value Change {
        n391 = event-data() -> ()  [unwired: 1 in, 1 out]
        n392 = Enqueue Element(queue=w1255, element=T1 {"DWF States"=enum."Quit", "Variant"=variant}) -> ()  [unwired: 2 in, 3 out]
      }
      event "Mode(N/T)": Value Change {
        n393 = event-data() -> ("NewVal"=w1256:bool)  [unwired: 1 in]
        n394 = Select(t=enum16{"Normal", "Turbo"}."Turbo" ("Mode"), s=w1256, f=enum16{"Normal", "Turbo"}."Normal" ("Mode")) -> (s? t:f=w1257:enum16{"Normal", "Turbo"})
        n395 = Bundle By Name(cluster=T1 {"DWF States"=enum."SetMode_", "Variant"=variant} ("element"), "Variant"=w1257) -> (w1260:T1)
        n396 = Enqueue Element(queue=w1262, element=w1260) -> ()  [unwired: 2 in, 3 out]
      }
      event "fConfig": Value Change {
        n397 = event-data() -> ()  [unwired: 1 in, 1 out]
        n398 = Enqueue Element(queue=w1264, element=T1 {"DWF States"=enum."fConfigurate", "Variant"=variant}) -> ()  [unwired: 2 in, 3 out]
      }
      event "Start": Value Change {
        n399 = event-data() -> ()  [unwired: 1 in, 1 out]
        n400 = Enqueue Element(queue=w1266, element=T1 {"DWF States"=enum."fStart", "Variant"=variant}) -> ()  [unwired: 2 in, 3 out]
      }
      event "TriggerPC": Value Change {
        n401 = event-data() -> ()  [unwired: 1 in, 1 out]
        n402 = Enqueue Element(queue=w1268, element=T1 {"DWF States"=enum."ManualTrigger", "Variant"=variant}) -> ()  [unwired: 2 in, 3 out]
      }
      event "Reset": Value Change {
        n403 = event-data() -> ()  [unwired: 1 in, 1 out]
        n404 = Enqueue Element(queue=w1270, element=T1 {"DWF States"=enum."Quit", "Variant"=variant}) -> ()  [unwired: 2 in, 3 out]
      }
      event "GetInfo": Value Change {
        n405 = event-data() -> ()  [unwired: 1 in, 1 out]
        n406 = Enqueue Element(queue=w1272, element=T1 {"DWF States"=enum."GetStatus", "Variant"=variant}) -> ()  [unwired: 2 in, 3 out]
      }
      event "CloseAll": Value Change {
        n407 = event-data() -> ()  [unwired: 1 in, 1 out]
        n408 = Enqueue Element(queue=w1274, element=T1 {"DWF States"=enum."CloseAll", "Variant"=variant}) -> ()  [unwired: 2 in, 3 out]
      }
      event "Close": Value Change {
        n409 = event-data() -> ()  [unwired: 1 in, 1 out]
        n410 = Enqueue Element(queue=w1276, element=T1 {"DWF States"=enum."Close", "Variant"=variant}) -> ()  [unwired: 2 in, 3 out]
      }
      event "Open": Value Change {
        n411 = event-data() -> ()  [unwired: 1 in, 1 out]
        n412 = Enqueue Element(queue=w1278, element=T1 {"DWF States"=enum."Open", "Variant"=variant}) -> ()  [unwired: 2 in, 3 out]
      }
      event "Enumerate": Value Change {
        n413 = event-data() -> ()  [unwired: 1 in, 1 out]
        n414 = Enqueue Element(queue=w1280, element=T1 {"DWF States"=enum."Enumerate", "Variant"=variant}) -> ()  [unwired: 2 in, 3 out]
      }
      event "SetStates_AO": Value Change {
        n415 = event-data() -> ()  [unwired: 1 in, 1 out]
        n416 = Bundle By Name(cluster=T27 {"Wait(s)"=0.0, "Run(s)"=0.0, "cRepeat"=1, "TriggerSource"=enum."None"} ("States"), "Wait(s)"=0.0, "Run(s)"=0.01, "cRepeat"=1) -> (w1288:T27)
        n417 = Bundle(0, "States"=w1288) -> (w1289:T28)  [unwired: 1 in]
        n418 = Bundle By Name(cluster=T1 {"DWF States"=enum."SetStates_AO", "Variant"=variant} ("element"), "Variant"=w1289) -> (w1282:T1)
        n419 = Enqueue Element(queue=w1290, element=w1282) -> ()  [unwired: 2 in, 3 out]
      }
      event "SetConfig_AO": Value Change {
        w1296 = 100.0  # 1/2 AI sample rate
        w1297 = T14 30 items=["DC"=0, "Sine"=1, "Square"=2, "Triangle"=3, "RampUp"=4, "RampDown"=5, "Noise"=6, "Custom"=30, "Play"=31] ("FUNC")
        n420 = event-data() -> ()  [unwired: 1 in, 1 out]
        n421 = Bundle By Name(cluster=T13 {"FUNC"=3, "Frequency(Hz)_AO"=512.0, "Amplitude(V)_AO"=1.0, "Phase(deg)_AO"=0.0, "Offset(V)_AO"=0.0, "rgdData"=[], "cData"=8192, "Symmetry"=0.0, "Enable"=TRUE, "Node"=enum."Carrier"}, "FUNC"=w1297, "Frequency(Hz)_AO"=w1296, "Amplitude(V)_AO"=1.0, "Phase(deg)_AO"=0.0, "Offset(V)_AO"=0.0, "Enable"=TRUE) -> (w1301:T13)
        n422 = Bundle(0, w1301) -> (w1292:cluster{i32, T13})  [unwired: 1 in]
        n423 = Bundle By Name(cluster=T1 {"DWF States"=enum."SetConfig_AO", "Variant"=variant} ("element"), "Variant"=w1292) -> (w1291:T1)
        n424 = Enqueue Element(queue=w1303, element=w1291) -> ()  [unwired: 2 in, 3 out]
      }
      event "SetEnable_AO": Value Change {
        w1305 = 0  # Channel_1
        n425 = event-data() -> ()  [unwired: 1 in, 1 out]
        n426 = Bundle("Channel_1"=w1305, TRUE) -> (w1306:cluster{"Channel_1":i32, bool})  [unwired: 1 in]
        n427 = Bundle By Name(cluster=T1 {"DWF States"=enum."SetChEnable_AO", "Variant"=variant} ("element"), "Variant"=w1306) -> (w1304:T1)
        n428 = Enqueue Element(queue=w1309, element=w1304) -> ()  [unwired: 2 in, 3 out]
      }
      event "SetTrigSrc_AO": Value Change {
        n429 = event-data() -> ()  [unwired: 1 in, 1 out]
        n430 = Bundle(0, "TriggerSource"=DWF_TrigSrc."PC") -> (w1312:cluster{i32, "TriggerSource":T9})  [unwired: 1 in]
        n431 = Bundle By Name(cluster=T1 {"DWF States"=enum."SetTriggerSource_AO", "Variant"=variant} ("element"), "Variant"=w1312) -> (w1311:T1)
        n432 = Enqueue Element(queue=w1315, element=w1311) -> ()  [unwired: 2 in, 3 out]
      }
      event "SetFuncData_AO": Value Change {
        w1326 = T14 30 items=["DC"=0, "Sine"=1, "Square"=2, "Triangle"=3, "RampUp"=4, "RampDown"=5, "Noise"=6, "Custom"=30, "Play"=31] ("FUNC")
        n433 = event-data() -> ()  [unwired: 1 in, 1 out]
        n434 = disable-structure shown="Disabled" {
          disable-tunnel: 1.0 ("Amplitude") -> [_ _]
          disable-tunnel: 32 ("NumRampPoints") -> [_ _]
          disable-tunnel: 2048 ("NumPoints") -> [_ w1331]
          disable-tunnel: [_ w1332] -> w1320
          frame Disabled {
          }
          frame Enabled {
            n435 = call-poly <vilib>:"Ramp Pattern.vi"("samples"=w1331) -> ("Ramp Pattern"=w1332:dbl[])  [unwired: 9 in, 1 out]
          }
        }
        n436 = Reverse 1D Array(array=w1320) -> (reversed array=w1321:dbl[])
        n437 = Build Array (concatenate)(w1320, w1321) -> (w1322:dbl[])
        n438 = Bundle By Name(cluster=T13 {"FUNC"=3, "Frequency(Hz)_AO"=512.0, "Amplitude(V)_AO"=1.0, "Phase(deg)_AO"=0.0, "Offset(V)_AO"=0.0, "rgdData"=[], "cData"=8192, "Symmetry"=0.0, "Enable"=TRUE, "Node"=enum."Carrier"}, "FUNC"=w1326, "rgdData"=w1322, "cData"=4096) -> (w1328:T13)
        n439 = Bundle(0, w1328) -> (w1318:cluster{i32, T13})  [unwired: 1 in]
        n440 = Bundle By Name(cluster=T1 {"DWF States"=enum."SetFuncData_AO", "Variant"=variant} ("element"), "Variant"=w1318) -> (w1316:T1)
        n441 = Enqueue Element(queue=w1330, element=w1316) -> ()  [unwired: 2 in, 3 out]
      }
      event "fStart_AO": Value Change {
        n442 = event-data() -> ()  [unwired: 1 in, 1 out]
        n443 = Bundle(0, 1) -> (w1335:cluster{i32, i32})  [unwired: 1 in]
        n444 = Bundle By Name(cluster=T1 {"DWF States"=enum."fStart_AO", "Variant"=variant} ("element"), "Variant"=w1335) -> (w1334:T1)
        n445 = Enqueue Element(queue=w1338, element=w1334) -> ()  [unwired: 2 in, 3 out]
      }
    }
    n446 = Or(x=w1218, y=w1216) -> (x .or. y?=w1217:bool)
  }
  n447 = Release Queue(queue=w4) -> ()  [unwired: 2 in, 3 out]
  n448 = Release Queue(queue=w25, error in (no error)=w23) -> (error out=w29:errorcluster)  [unwired: 1 in, 2 out]
  n449 = Release Queue(queue=w30, error in (no error)=w29) -> (error out=w27:errorcluster)  [unwired: 1 in, 2 out]
  n450 = Merge Errors(w16, w27) -> (w17:errorcluster)
  n451 = Release Queue(queue=w28, error in (no error)=w17) -> (error out=w22:errorcluster)  [unwired: 1 in, 2 out]
  n452 = call <vilib>:"General Error Handler.vi"("type of dialog (OK msg:1)"=w21, "error in (no error)"=w22, "[exception action] (none:0)"=w20, "[exception code]"=w19) -> ()  [unwired: 7 in, 5 out]
